vi "FrontPanel.vi"() -> ()   [LabVIEW 2013]
doc: "This VI controls the blindpanel type GHS-2T-1T-700 for a CryoFree DR. Automatization control is embedded in the blindpanel. Keys can be manipulated from within this VI."
uses:
  Write to PGSQL/FP to PGSQL/Typedefs/FP-cluster.ctl
  Lib/Lib.llb/ErrCodeStatusLkup.vi
  Lib/Lib.llb/Pfeiffer Vacuum.lvlib
  Lib/Lib.llb/MView.lvlib
  Lib/Lib.llb/Busy PopUp.lvlib
panel:
  out "VIRef":T1 {"Array DataType" format="%.0x"; "WaveForm Type" format="%.0x"; "RefNum Type" format="%.0x"; "DataType" format="%.0x"}
  out "ControlNames":string[](array[string])
  in  "Toolbar":enum32{"Page 1", "Page 2"}(tab)
  in  "Load config":bool
  in  "Save config":bool
  in  "Start":bool
  in  "Stop":bool
  out "V":string
  out "PT2 Data":dbl[](array[numeric])
  in  "Restart PT on Error?":bool
  in  "Attempts":u16=6
  in  "Time delay":u16=60 format="%.0f s"
  out "Error Log":string[][](table)
  in  "Error panel":enum32{"Page 1"}(tab)
  out "PT2 error":errorcluster
  out "MG error":errorcluster
  out "PT1 error":errorcluster
  out "FP error":errorcluster
  out "PT1 Data":dbl[](array[numeric])
  in  "Main Panel":enum32{"Page 1", "Page 2"}(tab)
  out "PC":sgl
  out "P1":sgl format="%.1f"
  out "P2":sgl format="%.1f"
  out "P3":sgl format="%.1f"
  out "P4":sgl format="%.1f"
  out "P5":sgl format="%.1f"
  out "P6":sgl format="%.1f"
  out "P7":sgl format="%.1f"
  out "Flow":sgl format="%#_4f"
  out "P5 alarm":bool
  out "Pstill (P8)":dbl format="%.1e"
  in  "Main Panel":T2(tab)
  out "String 2":string
  out "String 4":string
  out "String":string
  out "String 3":string
  out "Mode":u16(ring) items=["AUTO MODE OFF", "START", "CONDENSING 3He", "CONDENSING 4He", "NORMAL CIRCULATION", "RECOVERY OF THE MIXTURE", "RECOVERY: BLOCKAGE OR OVERPRESSURE"]
  out "FLOW":sgl format="%#_3f"
  out "P5":sgl
  out "P4":sgl
  out "P3":sgl
  out "P1":sgl
  out "P2":sgl
  out "3He":sgl(slide) min=0 max=2 scale=0.0..2000.0 scale format="%.2f"
  out "4He":sgl(slide) min=0 max=2 scale=0.0..2000.0 scale format="%.2f"
  out "Panel ID":string
  in  "FP type":enum32{"OLD", "NEW"}(tab)
  in  "Buttons":T3
  out "LEDs":T4
  in  "Buttons 2":T3
  out "LEDs 2":T5
  out "PC":sgl
  in  "PT Start 2":bool
  in  "PT_stop 2":bool
  in  "PT2 Plots Select":T6
  out "PT2 Status":cluster{"Time":dbl[], "Value":dbl[]}[](graph)
  in  "PT_ResetValues 2":bool
  out "PT Error Code 2":i32 caption="PT Error Code"
  out "PT Error 2":string="NO ERROR" caption="PT Error"
  out "P High":cluster{dbl, dbl, dbl, dbl}(slide) scale=150.0..450.0
  out "P Low":cluster{dbl, dbl, dbl, dbl}(slide) scale=0.0..300.0
  out "P_avg 2":cluster{"Low":dbl, "High":dbl} caption="Average pressure"
  out "Helium":cluster{dbl, dbl, dbl, dbl}(slide) scale=0.0..95.0
  out "Water In":cluster{dbl, dbl, dbl, dbl}(slide) scale=0.0..35.0
  out "Water Out":cluster{dbl, dbl, dbl, dbl}(slide) scale=0.0..60.0
  out "PT Status":u16(ring) items=["Compressor OFF", "Compressor ON", ""]
  out "Motor":cluster{dbl, dbl}(slide) scale=0.0..30.0
  out "Oil":cluster{dbl, dbl, dbl, dbl}(slide) scale=0.0..60.0
  in  "PT1 Plots Select":T6
  out "PT1 Status 2":cluster{"Time":dbl[], "Value":dbl[]}[](graph)
  out "P Low":cluster{dbl, dbl, dbl, dbl}(slide) scale=0.0..300.0
  out "P High":cluster{dbl, dbl, dbl, dbl}(slide) scale=150.0..450.0
  out "P_avg":cluster{"Low":dbl, "High":dbl} caption="Average pressure"
  out "Motor":cluster{dbl, dbl}(slide) scale=0.0..30.0
  out "Oil":cluster{dbl, dbl, dbl, dbl}(slide) scale=0.0..60.0
  out "Helium":cluster{dbl, dbl, dbl, dbl}(slide) scale=0.0..95.0
  out "Water Out":cluster{dbl, dbl, dbl, dbl}(slide) scale=0.0..60.0
  out "Water In":cluster{dbl, dbl, dbl, dbl}(slide) scale=0.0..35.0
  out "PT Error Code":i32
  out "PT Error":string="NO ERROR"
  in  "PT_ResetValues":bool
  in  "PT Start":bool
  in  "PT_stop":bool
  out "PT Status":u16(ring) items=["Compressor OFF", "Compressor ON", ""]
  in  "MG Plots Select":T6
  in  "FP Plots Select":T6
  out "MaxiGauge":cluster{"Time":dbl[], "Value":dbl[]}[](graph)
  out "Front Panel":cluster{"Time":dbl[], "Value":dbl[]}[](graph)
  in  "Boolean 2":bool
  out "PT2 port":u16
  out "PT1 port":u16
  out "MG port":refnum<visa-resource-name>="COM4" caption="Port number"
  out "FP port":refnum<visa-resource-name>="COM3" caption="Port number"
  out "ForceSave":bool
  in  "Button":u8
  out "SetControl":T7
  in  "S2":enum32{"Page 1"}(tab)
  in  "Reset Error 2":bool
  in  "S1":enum32{"Page 1"}(tab)
  in  "Reset Error":bool
  out "Cur Path":path
  in  "Side Panel":enum32{"Main", "Settings", "Advanced"}(tab)=enum."Settings"
  out "Maxigauge ID":string caption="ID"
  out "Panel response":string
  out "Sensors Status":T8={"String 8"="OK", "String 9"="OK", "String 10"="OK", "String 11"="OK", "String 12"="OK", "String 13"="OK"}
  in  "ADC scaling":T9={"P1"=2500.0, "P2"=2500.0, "P3"=2500.0, "P4"=2500.0, "P5"=2500.0, "P6"=2500.0, "P7"=2500.0, "Flow meter"=682.0, "PC"=10000.0} caption="Front panel ADC scaling factors" {"Flow meter" format="%#.4f"}
  in  "REC Settings":T10={"P6 low"=20, "P6 high"=1000, "P7 low"=20}
  in  "NCP5B Settings":cluster{"P6 low":u16}={"P6 low"=20}
  in  "NCP5 Settings":T10={"P6 low"=20, "P6 high"=1000, "P7 low"=20}
  in  "S1&2 Settings":cluster{"Enum":enum16{"OFF", "ON"}}
  in  "P5 Settings":cluster{"P6 low":u16, "P6 high":u16}={"P6 low"=20, "P6 high"=1000}
  out "REC limits":T11={"P5 warn"=20, "P5 rec"=20, "P5 res"=20}
  out "NCP5B limits":cluster{"P5 NC4":u16}={"P5 NC4"=20}
  out "NCP5 limits":T12={"P5 NC1"=20, "P5 NC2"=20, "P5 NC3"=20}
  out "S1&2 limits":cluster{"S1&S2":enum16{"OFF", "ON"}}
  out "P5 limits":cluster{"P5 C1":u16, "P5 C2":u16}={"P5 C1"=20, "P5 C2"=20}
  in  "P6&7 Settings":T13={"P6 low"=20, "P6 high"=1600, "P7 low"=20, "P7 high"=1610}
  out "P6&7 limits":T13={"P6 low"=20, "P6 high"=20, "P7 low"=20, "P7 high"=20}
  in  "SET VALUES":bool
  out "MG pressures":T14 {"Channel 1" format="%-7.2e mbar"; "Channel 1" format="%-7.2e mbar"; "Channel 1" format="%-7.2e mbar"; "Channel 1" format="%-7.2e mbar"; "Channel 1" format="%-7.2e mbar"; "Channel 1" format="%-7.2e mbar"}
  out "Cluster":T15={"String 2"="\"\"", "String 3"="", "String 4"="", "String 5"="", "String 6"="", "String 7"=""}
  in  "Log Options":T16={"Plot data "=TRUE, "Every1"=1.0, "Save to log"=TRUE, "Every  2"=1.0, "AVS_Path 2"=path "C:/LC Data/Data", "AVS_FName"="logFP", "Filename suffix"="_%Y-%m-%d-%H-%M-%S", "NewFevery"=7, "Time Units"=enum."Days", "Date Format"="%Y-%m-%d %H:%M:%S", "Averages"=4} caption="Data Logging \nOptions" {"Every  2" format="%#_g min"; "Every1" format="%#_g min"}
  in  "Configuration":T17={"FP port number"="COM3", "MG port number"="COM4", "PT1 Enabled?"=FALSE, "MG  channel P8"=65535, "Stop auto recovery if still is empty"=FALSE, "PT1 port number"="COM2", "MG Enabled?"=TRUE, "PT1 Address"=16, "S1 Enabled?"=FALSE, "S1 port"="COM2", "S2 Enabled?"=FALSE, "S2 port"="COM2", "Device address S1"=1, "Device address S2"=2, "PT1 Bauds"=115200, "PT2 Enabled?"=FALSE, "PT2 port number"="COM2", "PT2 Address"=16, "PT2 Bauds"=115200, "FP baud rate"=9600} {"PT2 Address" min=16 max=126 step=1; "MG  channel P8" items=["Channel 1", "Channel 2", "Channel 3", "Channel 4", "Channel 5", "Channel 6"]; "PT1 Address" min=16 max=126 step=1}
  in  "Type":enum32{"Wet", "CF"}(radio)=enum."CF"
  in  "Panel Layout":enum32{"OLD", "NEW"}(ring)=enum."NEW"
  out "RAW ADC Values 2":dbl[](array[numeric]) caption="Converted ADC Values"
  in  "SendCMD":bool caption="Send"
  out "Response":string
  in  "Command":string
  out "SP reached? 2":bool
  in  "Cond1":bool
  in  "Delay Time":u32=30 caption="For a time delay of" format="%.0f min"
  in  "MG  channel":u16(ring)=65535 caption="MaxiGauge" items=["Channel 1", "Channel 2", "Channel 3", "Channel 4", "Channel 5", "Channel 6"]
  out "SP reached? 3":bool
  in  "P threshold":dbl=0.0005 caption="<" format="%#_2g mbar"
  in  "Cond2":bool
  out "SP reached?":bool
  out "Delay Timer":u32=10 caption="Timer" format="%<%M:%S>t"
  in  "EnableAutoCond":bool caption="Start"
  out "VI path":string
  out "RAW ADC Values":i32[](array[numeric])
  in  "Autoconf":bool caption="Autoconfigure"
  out "MG Data":dbl[](array[numeric]) format="%.3e"
  out "FP Data":sgl[](array[numeric]) format="%.2f"
  out "FP Status bits":u32[](array[numeric])
  out "Attempts Counter":u16
  # "Error log"
  # "Front panel status"
  # "MaxiGauge status"
  # "Pulse Tube 1 status"
  # "Pulse Tube 2 status"
  # "Leiden Cryogenics"
  # "to \nair"
  # "N.C."
  # "from\novc"
  # "from\nivc"
  # "from still"
  # "to 3He\nin-1"
  # "to 3He\nin-2"
  # "P8"
  # "AUX 1"
  # "BYPASS"
  # "MIXTURE\nCOMPRESSOR"
  # "M2"
  # "P6"
  # "M3"
  # "M1"
  # "AUX PORT-1"
  # "P7"
  # "TRAP"
  # "AUX TRAP"
  # "To \nAir"
  # "From\nIVC"
  # "From Still"
  # "To 3He\nin-1"
  # "To 3He\nin-2"
  # "To \nAir"
  # "N.C."
  # "from\novc"
  # "from\nivc"
  # "from still"
  # "to 3He\nin-1"
  # "to 3He\nin-2"
  # "Leiden Cryogenics"
  # "to \nair"
  # "N.C."
  # "from\novc"
  # "from\nivc"
  # "from still"
  # "to 3He\nin-1"
  # "to 3He\nin-2"
  # "P8"
  # "M2"
  # "P6"
  # "M3"
  # "TRAP"
  # "AUX TRAP"
  # "M1"
  # "AUX PORT-1"
  # "P7"
  # "AUX 1"
  # "To \nAir"
  # "From\nIVC"
  # "From Still"
  # "To 3He\nin-1"
  # "to 3He\nin-1"
  # "To 3He\nin-2"
  # "to \nair"
  # "N.C."
  # "from\novc"
  # "from\nivc"
  # "from still"
  # "to 3He\nin-2"
  # "Pulse Tube 1"
  # "Pulse Tube 2"
  # "Front Panel"
  # "MaxiGauge"
  # "Turbo2 (S2)"
  # "Turbo1 (S1)"
  # "MaxiGauge"
  # "#"
  # "NAME"
  # "PRESSURE"
  # "STATUS"
  # "1"
  # "2"
  # "3"
  # "4"
  # "5"
  # "6"
  # "Automatic mode pressure limits"
  # "Warning: These values influence the operation of the GHS in automatic mode. Please refer to the operation manual and consult with Leiden Cryogenics before changing them."
  # "NAME"
  # "FW"
  # "NEW"
  # "DESCRIPTION"
  # "Stop condensing 4He"
  # "Stop recovering 4He"
  # "Stop condensing 3He"
  # "Stop recovering 3He"
  # "Condensing->open 12"
  # "Condensing->close 9/12"
  # "Condensing->run S1&S2"
  # "NC->open second line"
  # "NC->start MC"
  # "NC->open aux. trap"
  # "NC->stop MC, close 7"
  # "All->P5 alarm"
  # "All->switch to recovery"
  # "All->reset"
  # "Front panel ADC scaling factors"
  # "Data Logging and Plotting"
  # "Front Panel"
  # "MaxiGauge"
  # "Pulse Tube 1"
  # "Pulse Tube 2"
  # "Turbo 1 (S1) (Pfeiffer HiPACE only)"
  # "Turbo2 (S2) (Pfeiffer HiPACE only)"
  # "Automatic condensing"
  # "Start condensing when"
  # "and wait"
  # "Send command to Front Panel"
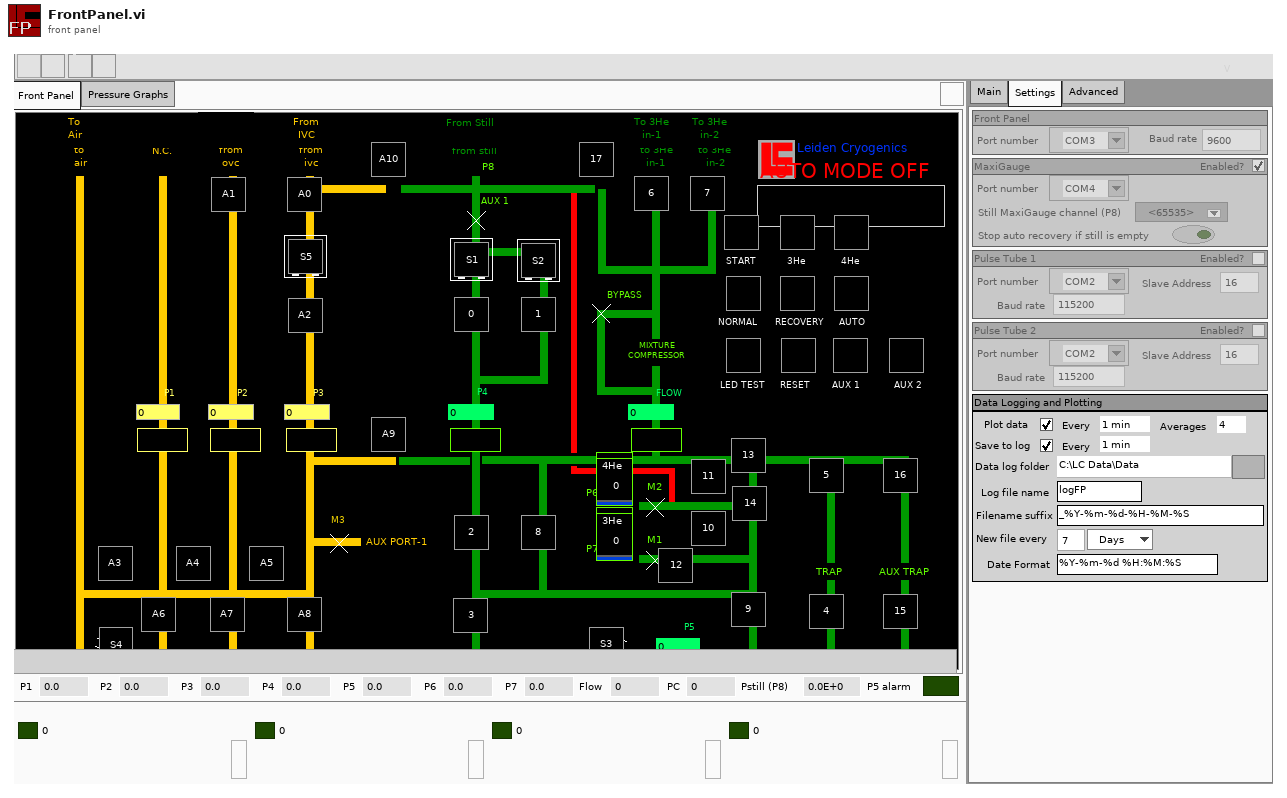
[diagram p1: front panel]
types:
  T1 = cluster{"Control Ref ID":refnum<vi>[], "Full Name":string[], "ClassID":enum16{"<Null>", "1", "2", "Generic", "Decoration", "Text", "Control", "ColorBox", "Boolean", "RefNum", "Variant", "Path", "ListBox", "Table", "Array", "Picture", "ActiveXContainer", "Numeric", "Digital", "NamedNumeric", "ColorRamp", "Slide", "GraphOrChart", "WaveformChart", "WaveformGraph", "IntensityChart", "IntensityGraph", "String", "IOName", "ComboBox", "Cluster", "Panel", "Knob", "NumWithScale", "Ring", "Enum", "GObject", "Plot", "Cursor", "NumericText", "Scale", "ColorScale", "GraphScale", "ColorGraphScale", "TypedRefNum", "OldKnobScale", "MCListbox", "MeasureData", "BVTag", "DAQName", "VISAName", "IVIName", "SlideScale", "TabControl", "Page", "TabArrayTabControl", "ConPane", "57", "58", "59", "60", "61", "62", "63", "64", "SubPanel", "TreeControl", "67", "68", "69", "70", "71", "72", "73", "74", "75", "SplitterBar"}[], "Short Name":string[], "DataType":enum8{"<Null>", "I8", "I16", "I32", "I64", "U8", "U16", "U32", "U64", "SGL", "DBL", "EXT", "CSG", "CDB", "CXT", "0x0F", "0x10", "0x11", "0x12", "0x13", "0x14", "Enum U8", "Enum U16", "Enum U32", "Enum U64", "SGL PQ", "DBL PQ", "EXT PQ", "CSG PQ", "CDB PQ", "CXT PQ", "0x1F", "0x20", "Boolean", "0x22", "0x23", "0x24", "0x25", "0x26", "0x27", "0x28", "0x29", "0x2A", "0x2B", "0x2C", "0x2D", "0x2E", "0x2F", "String", "0x31", "Path", "Pict", "0x34", "0x35", "0x36", "DAQ", "0x38", "0x39", "0x3A", "0x3B", "0x3C", "0x3D", "0x3E", "0x3F", "Array", "0x41", "0x42", "0x43", "0x44", "0x45", "0x46", "0x47", "0x48", "0x49", "0x4A", "0x4B", "0x4C", "0x4D", "0x4E", "0x4F", "Cluster", "0x51", "0x52", "Variant", "Waveform", "0x55", "0x56", "0x57", "0x58", "0x59", "0x5A", "0x5B", "0x5C", "0x5D", "0x5E", "0x5F", "0x60", "0x61", "0x62", "0x63", "0x64", "0x65", "0x66", "0x67", "0x68", "0x69", "0x6A", "0x6B", "0x6C", "0x6D", "0x6E", "0x6F", "Refnum"}[], "RefNum Type":enum8{"Generic", "Datalog File Refnum", "Byte Stream File Refnum", "Device Refnum", "Occurence Refnum", "TCP Connection Refnum", "VISA Refnum (Obsolete)", "Automation Renum", "VI Server Refnum", "Menu Refnum", "IVI Refnum (Obsolete)", "IMAQ Session", "0x0C", "Datasocket Refnum", "VISA Resource", "IVI Logical Name", "UDP Connection Refnum", "Notifier Refnum", "Queue Refnum", "IrDA Refnum", "Hardware Plugin Refnum", "Hardware Plugin Tag Refnum", "DAQmx Refnum", "Event Registration Refnum", ".NET Refnum", "User Event Refnum", "0x1A", "Event Callback", "0x1C", "0x1D", "Only Used Internal to LabVIEW", "Bluetooth", "Data Value References", "RT FIFO", "TDM Streaming"}[], "WaveForm Type":enum8{"<Not a Waveform Type>", "0x01", "Analog 16-bit signed", "Analog Double-Precision", "0x04", "Analog Single Precision", "Timestamp", "Digital Data", "Digital Waveform", "Dynamic Data", "Analog Extended-Precision", "Analog 8-bit unsigned", "Analog 16-bit unsigned", "Analog 32-bit unsigned", "Analog 8-bit signed", "Analog 32-bit signed", "Analog Complex Single-Precision", "Analog Complex Double-Precision", "Analog Complex Extended Precision", "Analog 64-bit signed", "Analog 64-bit unsigned"}[], "Parent":i32[], "Array DataType":enum8{"<Null>", "I8", "I16", "I32", "I64", "U8", "U16", "U32", "U64", "SGL", "DBL", "EXT", "CSG", "CDB", "CXT", "0x0F", "0x10", "0x11", "0x12", "0x13", "0x14", "Enum U8", "Enum U16", "Enum U32", "Enum U64", "SGL PQ", "DBL PQ", "EXT PQ", "CSG PQ", "CDB PQ", "CXT PQ", "0x1F", "0x20", "Boolean", "0x22", "0x23", "0x24", "0x25", "0x26", "0x27", "0x28", "0x29", "0x2A", "0x2B", "0x2C", "0x2D", "0x2E", "0x2F", "String", "0x31", "Path", "Pict", "0x34", "0x35", "0x36", "DAQ", "0x38", "0x39", "0x3A", "0x3B", "0x3C", "0x3D", "0x3E", "0x3F", "Array", "0x41", "0x42", "0x43", "0x44", "0x45", "0x46", "0x47", "0x48", "0x49", "0x4A", "0x4B", "0x4C", "0x4D", "0x4E", "0x4F", "Cluster", "0x51", "0x52", "Variant", "Waveform", "0x55", "0x56", "0x57", "0x58", "0x59", "0x5A", "0x5B", "0x5C", "0x5D", "0x5E", "0x5F", "0x60", "0x61", "0x62", "0x63", "0x64", "0x65", "0x66", "0x67", "0x68", "0x69", "0x6A", "0x6B", "0x6C", "0x6D", "0x6E", "0x6F", "Refnum"}[], "Owning VI":refnum<vi>[], "Active?":bool[]}
  T2 = enum32{"Front Panel", "PulseTube", "Pressure Graphs"}
  T3 = cluster{"baux2":bool, "bBypass":bool, "b15":bool, "b16":bool, "NC 0":bool, "baux1":bool, "b4":bool, "NC 1":bool, "b5":bool, "breset":bool, "NC 2":bool, "b9":bool, "b14":bool, "NC 3":bool, "b13":bool, "bledtest":bool, "NC 4":bool, "b12":bool, "b10":bool, "NC 5":bool, "b11":bool, "bA0":bool, "NC 9":bool, "b7":bool, "bS3":bool, "NC 12":bool, "b6":bool, "b17":bool, "NC 13":bool, "b8":bool, "b1":bool, "NC 14":bool, "bS2":bool, "b3":bool, "NC 15":bool, "b2":bool, "b0":bool, "NC 16":bool, "bS1":bool, "bA9":bool, "NC 17":bool, "bA8":bool, "bA2":bool, "NC 6":bool, "bs5":bool, "bA10":bool, "NC 7":bool, "bstart":bool, "bA5":bool, "NC 8":bool, "bA7":bool, "bA1":bool, "NC 10":bool, "bauto":bool, "bA4":bool, "NC 11":bool, "bA6":bool, "bS4":bool, "NC 18":bool, "bA3":bool, "b3he":bool, "b4he":bool, "bnorm":bool, "brecov":bool}
  T4 = cluster{"COMPR/AUX 2":bool, "BYPASS":bool, "15":bool, "16":bool, "NC 0":bool, "AUX 1":bool, "4":bool, "NC 1":bool, "5":bool, "RESET":bool, "NC 2":bool, "9":bool, "14":bool, "NC 3":bool, "13":bool, "LED TEST":bool, "NC 4":bool, "12":bool, "10":bool, "NC 5":bool, "11":bool, "A0":bool, "NC 12":bool, "7":bool, "S3":bool, "NC 13":bool, "6":bool, "17":bool, "NC 14":bool, "8":bool, "1":bool, "NC 15":bool, "S2":bool, "3":bool, "NC 16":bool, "2":bool, "0":bool, "NC 17":bool, "S1":bool, "A9":bool, "NC 6":bool, "A8":bool, "A2":bool, "NC 7":bool, "S5":bool, "A10":bool, "NC 8":bool, "START":bool, "A5":bool, "NC 9":bool, "A7":bool, "A1":bool, "NC 10":bool, "AUTO":bool, "A4":bool, "NC 11":bool, "A6":bool, "S4":bool, "NC 18":bool, "A3":bool, "3He":bool, "4He":bool, "NORMAL":bool, "RECOVERY":bool, "PT STATUS":bool}
  T5 = cluster{"COMPR/AUX 2":bool, "BYPASS":bool, "15":bool, "16":bool, "AUX 1":bool, "AUX 1":bool, "4":bool, "AUX 2":bool, "5":bool, "RESET":bool, "AUX 3":bool, "9":bool, "14":bool, "NC 3":bool, "13":bool, "LED TEST":bool, "NC 4":bool, "12":bool, "10":bool, "NC 5":bool, "11":bool, "A0":bool, "NC 12":bool, "7":bool, "S3":bool, "NC 13":bool, "6":bool, "17":bool, "NC 14":bool, "8":bool, "1":bool, "NC 15":bool, "S2":bool, "3":bool, "NC 16":bool, "2":bool, "0":bool, "NC 17":bool, "S1":bool, "A9":bool, "NC 6":bool, "A8":bool, "A2":bool, "NC 7":bool, "S5":bool, "A10":bool, "NC 8":bool, "START":bool, "A5":bool, "NC 9":bool, "A7":bool, "A1":bool, "NC 10":bool, "AUTO":bool, "A4":bool, "NC 11":bool, "A6":bool, "S4":bool, "NC 18":bool, "A3":bool, "3He":bool, "4He":bool, "NORMAL":bool, "RECOVERY":bool, "PT STATUS":bool}
  T6 = cluster{"Boolean":bool, "Boolean 2":bool, "Boolean 3":bool, "Boolean 4":bool, "Boolean 5":bool, "Boolean 6":bool, "Boolean 7":bool, "Boolean 8":bool}
  T7 = cluster{"Name":string, "Scalar":string, "Array":string[][]}
  T8 = cluster{"String 8":string, "String 9":string, "String 10":string, "String 11":string, "String 12":string, "String 13":string}
  T9 = cluster{"P1":dbl, "P2":dbl, "P3":dbl, "P4":dbl, "P5":dbl, "P6":dbl, "P7":dbl, "Flow meter":dbl, "PC":dbl}
  T10 = cluster{"P6 low":u16, "P6 high":u16, "P7 low":u16}
  T11 = cluster{"P5 warn":u16, "P5 rec":u16, "P5 res":u16}
  T12 = cluster{"P5 NC1":u16, "P5 NC2":u16, "P5 NC3":u16}
  T13 = cluster{"P6 low":u16, "P6 high":u16, "P7 low":u16, "P7 high":u16}
  T14 = cluster{"Channel 1":dbl, "Channel 1":dbl, "Channel 1":dbl, "Channel 1":dbl, "Channel 1":dbl, "Channel 1":dbl}
  T15 = cluster{"String 2":string, "String 3":string, "String 4":string, "String 5":string, "String 6":string, "String 7":string}
  T16 = cluster{"Plot data ":bool, "Every1":dbl, "Save to log":bool, "Every  2":dbl, "AVS_Path 2":path, "AVS_FName":string, "Filename suffix":string, "NewFevery":u32, "Time Units":enum16{"Minutes", "Hours", "Days"}, "Date Format":string, "Averages":i32}
  T17 = cluster{"FP port number":refnum<visa-resource-name>, "MG port number":refnum<visa-resource-name>, "PT1 Enabled?":bool, "MG  channel P8":u16, "Stop auto recovery if still is empty":bool, "PT1 port number":refnum<visa-resource-name>, "MG Enabled?":bool, "PT1 Address":u8, "S1 Enabled?":bool, "S1 port":refnum<visa-resource-name>, "S2 Enabled?":bool, "S2 port":refnum<visa-resource-name>, "Device address S1":u8, "Device address S2":u8, "PT1 Bauds":u32, "PT2 Enabled?":bool, "PT2 port number":refnum<visa-resource-name>, "PT2 Address":u8, "PT2 Bauds":u32, "FP baud rate":u32}
  T18 = cluster{"error":bool, "code":i32, "source":string}
  T19 = cluster{"Dict. Var":u16, "Description":string, "Values":i32[]}[]
  T20 = cluster{"[3]":dbl, "[3]":dbl, "[3]":dbl, "Values[3] 2":dbl}
  T21 = cluster{"[1]":dbl, "[1]":dbl, "[1]":dbl, "Values[1] 2":dbl}
  T22 = cluster{"Values[0]":dbl, "Values[0]":dbl, "Values[0]":dbl, "Values[0] 2":dbl}
  T23 = cluster{"error":bool, "code":i32, "error source":string}
  T24 = cluster{"sensor status info[0]":string, "sensor status info[1]":string, "sensor status info[2]":string, "sensor status info[3]":string, "sensor status info[4]":string, "sensor status info[5]":string}
  T25 = cluster{"Filterred[0]":dbl, "Filterred[1]":dbl, "Filterred[2]":dbl, "Filterred[3]":dbl, "Filterred[4]":dbl, "Filterred[5]":dbl}
  T26 = typedef "FP-cluster.ctl" = cluster{"FP Data":sgl[], "MG Data":dbl[], "PT Data":dbl[], "FP Status Bits":u32[], "Mode":u16}
  T27 = cluster{"FP Data[0]":sgl, "FP Data[1]":sgl, "FP Data[2]":sgl, "FP Data[3]":sgl, "FP Data[4]":sgl, "FP Data[5]":sgl, "FP Data[6]":sgl, "FP Data[7]":sgl, "FP Data[8]":sgl}
  T28 = enum32{"Page Enabled", "Page Disabled", "Page Disabled & Grayed"}
  T29 = enum32{"invalid app kind", "Development System", "Run Time System", "Student Edition", "Embedded LabVIEW", "Evaluation", "Custom"}
  T30 = cluster{"array of 4 x 16 bit unsigned[0]":u16, "array of 4 x 16 bit unsigned[1]":u16, "array of 4 x 16 bit unsigned[2]":u16, "array of 4 x 16 bit unsigned[3]":u16}
  T31 = cluster{"array of 2 x 16 bit unsigned[0]":u16, "array of 2 x 16 bit unsigned[1]":u16}
  T32 = cluster{"array of 3 x 16 bit unsigned[0]":u16, "array of 3 x 16 bit unsigned[1]":u16, "array of 3 x 16 bit unsigned[2]":u16}
  T33 = cluster{"Array[0]":string, "Array[1]":string, "Array[2]":string, "Array[3]":string, "Array[4]":string, "Array[5]":string}
  T34 = typedef "LVRectTypeDef.ctl" = cluster{"Left":i16, "Top":i16, "Right":i16, "Bottom":i16}
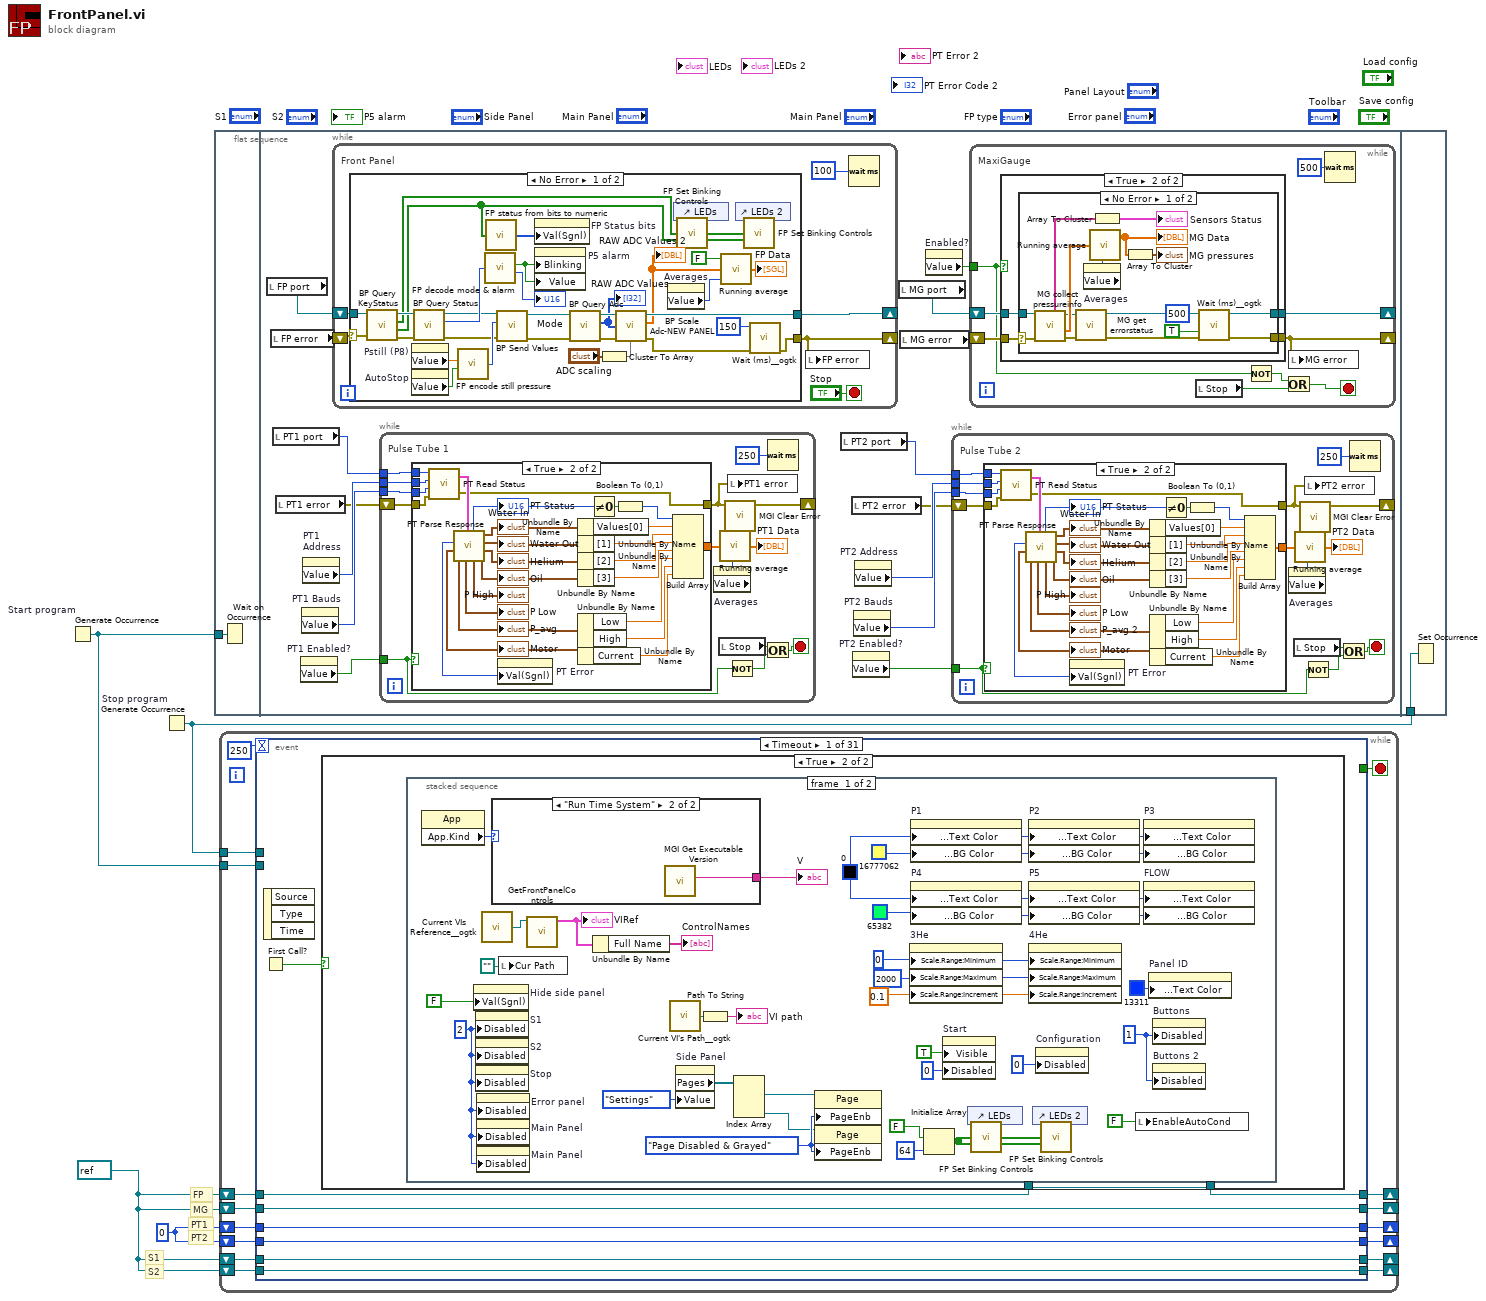
[diagram p0: block diagram]
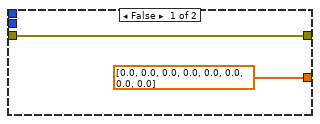
[diagram p2: hidden frame]
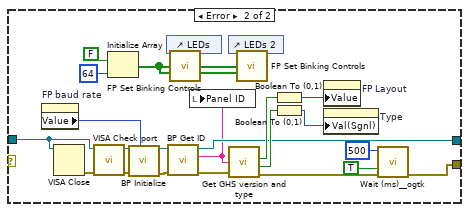
[diagram p3: hidden frame]
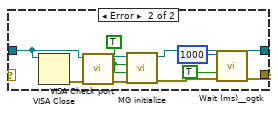
[diagram p5: hidden frame]
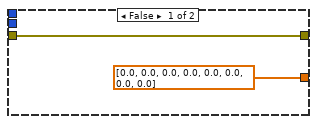
[diagram p6: hidden frame]
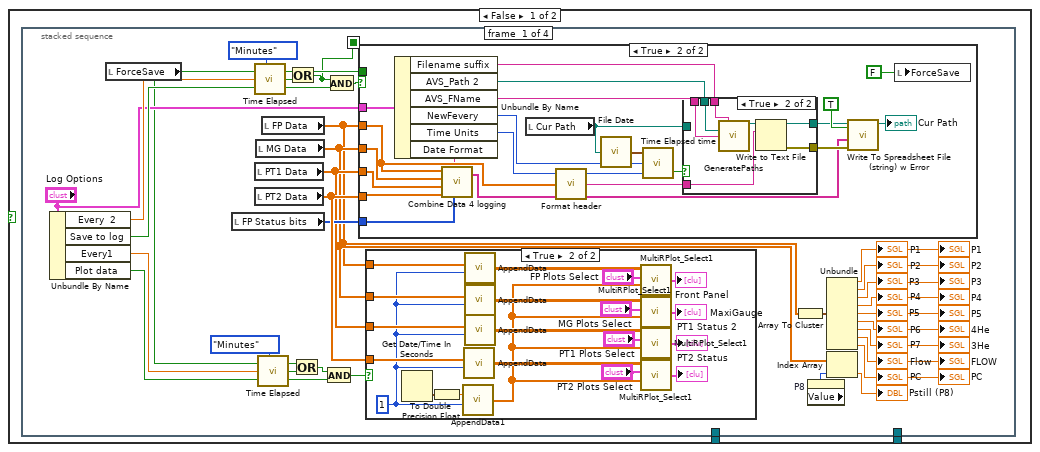
[diagram p7: hidden frame]
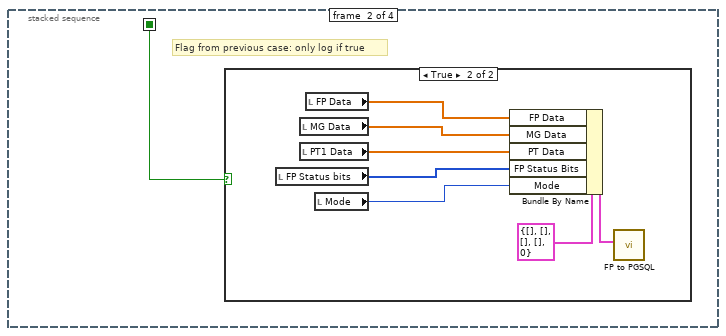
[diagram p11: hidden frame]
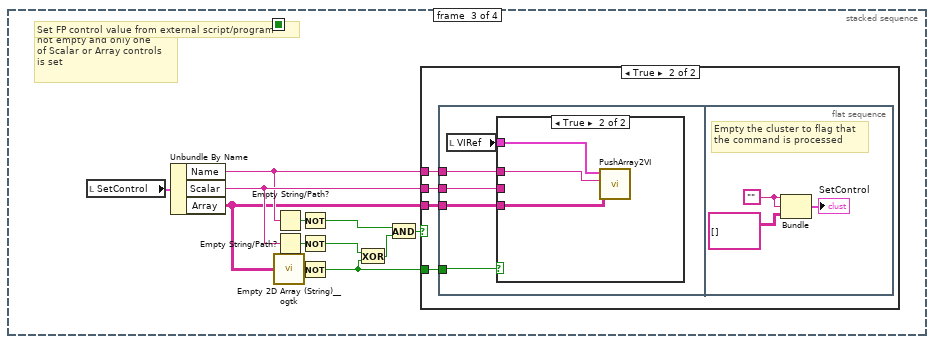
[diagram p13: hidden frame]
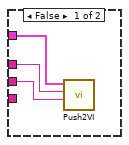
[diagram p15: hidden frame]
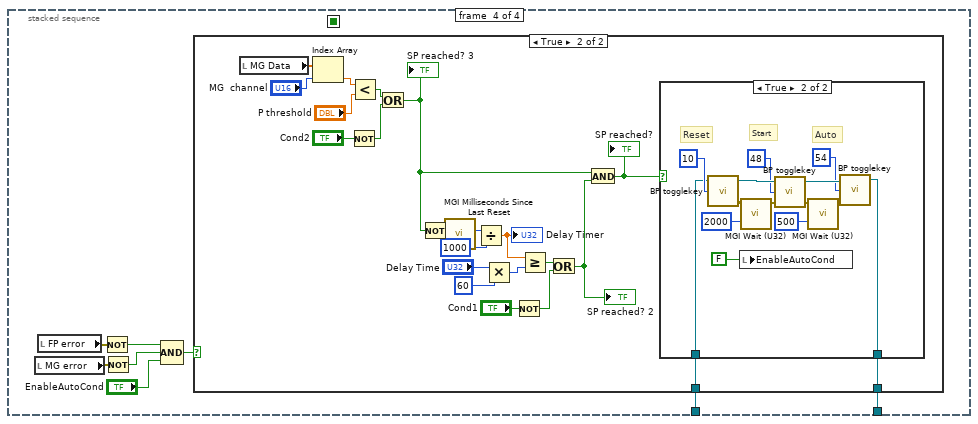
[diagram p16: hidden frame]
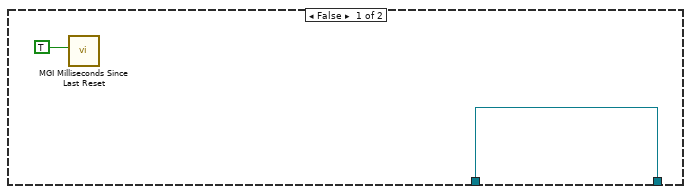
[diagram p17: hidden frame]
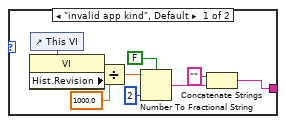
[diagram p19: hidden frame]
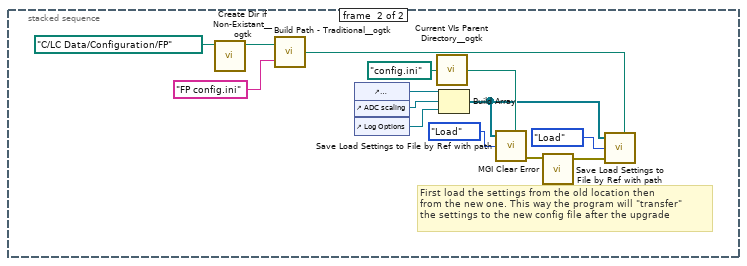
[diagram p20: hidden frame]
diagram:
  w1 = u8 0 ("x+1")
  w2 = refnum<visa-resource-name> refnum ("PT port")
  # "S2"
  # "S1"
  # "MG"
  # "PT1"
  # "PT2"
  # "FP"
  n1 = Generate Occurrence "Start program"() -> (w4:refnum<k4>)
  n2 = Generate Occurrence "Stop program"() -> (w3:refnum<k4>)
  n3 = flat-sequence {
    tunnel: w4 -> [w5]
    tunnel: w3 -> [w204]
    frame #0 {
      n4 = Wait on Occurrence(2:w5) -> ()  [unwired: 2 in, 1 out]
    }
    frame #1 {
      n5 = local read "FP port"() -> (w11:refnum<visa-resource-name>)
      n6 = local read "FP error"() -> (w16:errorcluster)
      n7 = local read "PT1 port"() -> (w7:u16)
      n8 = local read "PT1 error"() -> (w8:errorcluster)
      n9 = property on="PT1 Enabled?" class="Bool (strict)"() -> ("Value"=w19:bool)  [unwired: 2 in, 2 out]
      n10 = property on="PT1 Bauds" class="DigNum (strict)"() -> ("Value"=w17:u32)  [unwired: 2 in, 2 out]
      n11 = property on="PT1 \nAddress" class="DigNum (strict)"() -> ("Value"=w20:u8)  [unwired: 2 in, 2 out]
      n12 = while {
        shift-right: [w66] -> _
        shift-left: w16 -> [w67]
        shift-right: [w64] -> _
        shift-left: w11 -> [w65]
        stop <- "Stop" stop-if-true
        # "Front Panel"
        n13 = case shown="No Error" w67 {
          selector: w67 -> [w97 _]
          tunnel: [w78 w111] -> w64
          tunnel: [w76 w109] -> w66
          tunnel: w65 -> [w98 w112]
          frame No Error {
            n14 = call "BP Query KeyStatus.vi"("error in"=w97, "FrontPanel port"=w98) -> ("error out"=w86:T18, "Button states"=w69:bool[], "Blinking States"=w70:bool[], "FrontPanel port"=w87:refnum<visa-resource-name>)  [unwired: 2 in]
            n15 = property on="Pstill (P8)" class="DigNum (strict)"() -> ("Value"=w88:dbl)  [unwired: 2 in, 2 out]
            n16 = property on="AutoStop" class="Bool (strict)"() -> ("Value"=w89:bool)  [unwired: 2 in, 2 out]
            n17 = call "BP Query Status.vi"("error in"=w86, "FrontPanel port"=w87) -> ("error out"=w91:T18, "status word (32 bit unsigned)"=w94:u32, "FrontPanel port"=w92:refnum<visa-resource-name>)  [unwired: 3 in]
            n18 = call "FP encode still pressure.vi"("Value 2"=w89, "Value"=w88) -> ("Numeric"=w93:u16)  [unwired: 4 in]
            n19 = call "FP decode mode & alarm.vi"("status word (32 bit unsigned)"=w94) -> ("Boolean"=w90:bool, "Numeric"=→"Mode":u32)  [unwired: 4 in]
            n20 = call "FP status from bits to numeric.vi"("FP Status bits"=w69) -> ("FP status number"=w96:u32[])  [unwired: 4 in]
            n21 = call "BP Send Values.vi"("error in"=w91, "value to send"=w93, "FrontPanel port"=w92) -> ("error out"=w80:T18, "FrontPanel port"=w81:refnum<visa-resource-name>)  [unwired: 3 in]
            n22 = property on="FP Status bits" class="Arr (strict)"("Val(Sgnl)"=w96) -> ()  [unwired: 2 in, 2 out]
            n23 = property on="P5 alarm" class="Bool (strict)"("Blinking"=w90, "Value"=w90) -> ()  [unwired: 2 in, 2 out]
            n24 = call "BP Query Adc.vi"("error in"=w80, "FrontPanel port"=w81) -> ("error out"=w77:T18, "array of 8(9) x 16 bit signed"=w72:i32[], "FrontPanel port"=w78:refnum<visa-resource-name>)  [unwired: 3 in]
            "RAW ADC Values" <- w72
            n25 = Cluster To Array(cluster="ADC scaling") -> (array=w79:dbl[])
            n26 = call "BP Scale Adc-NEW PANEL.vi"("input array scaling factors,8(9) x 16 bit uint"=w79, "input array 8(9) x 16bit uint"=w72) -> ("output array 8(9) x single prec. incl flow"=w71:sgl[])  [unwired: 4 in, 1 out]
            "RAW ADC Values 2" <- w71
            n27 = property on="Averages" class="DigNum (strict)"() -> ("Value"=w85:i32)  [unwired: 2 in, 2 out]
            n28 = control-ref of="LEDs"() -> (w74:refnum<vi>)
            n29 = call "FP Set Binking Controls.vi"("Cluster in"=w74, "Array of blinking states"=w70, "Array of relais states"=w69) -> ()  [unwired: 13 in]
            n30 = call "Running average.vi"("Window Size"=w85, "New values"=w71, "Filter Zeroes? (T)"=FALSE) -> ("Filterred"=→"FP Data":dbl[])  [unwired: 1 in]
            n31 = control-ref of="LEDs 2"() -> (w73:refnum<vi>)
            n32 = call "FP Set Binking Controls.vi"("Cluster in"=w73, "Array of blinking states"=w70, "Array of relais states"=w69) -> ()  [unwired: 13 in]
            n33 = call "Wait (ms)__ogtk.vi"("error in (no error)"=w77, "milliseconds to wait"=u32 150) -> ("error out"=w76:errorcluster)  [unwired: 8 in, 1 out]
          }
          frame Error {
            n34 = property on="FP baud rate" class="DigNum (strict)"() -> ("Value"=w104:u32)  [unwired: 2 in, 2 out]
            n35 = VISA Close(VISA resource name=w112) -> (error out=w121:errorcluster)  [unwired: 1 in]
            n36 = call "VISA Check port.vi"("error in (no error)"=w121, "VISA Resource Name in"=w112) -> ("error out"=w120:errorcluster, "VISA Resource Name out"=w119:refnum<visa-resource-name>)  [unwired: 8 in]
            n37 = Initialize Array(FALSE, 64 ("dimension size")) -> (w99:bool[])
            n38 = call "BP Initialize.vi"("FP baud rate"=w104, "error in (no error)"=w120, "FrontPanel port"=w119) -> ("error out"=w118:errorcluster, "FrontPanel port"=w117:refnum<visa-resource-name>)  [unwired: 4 in]
            n39 = control-ref of="LEDs"() -> (w101:refnum<vi>)
            n40 = call "BP Get ID.vi"("error in (no error)"=w118, "FrontPanel port"=w117) -> ("error out"=w106:errorcluster, "Device ID string"=w110:string, "FrontPanel port"=w111:refnum<visa-resource-name>)  [unwired: 6 in, 1 out]
            n41 = call "FP Set Binking Controls.vi"("Cluster in"=w101, "Array of blinking states"=w99, "Array of relais states"=w99) -> ()  [unwired: 13 in]
            n42 = local write "Panel ID"(w110) -> ()
            n43 = control-ref of="LEDs 2"() -> (w100:refnum<vi>)
            n44 = call "Get GHS version and type.vi"("ID string"=w110, "error in (no error)"=w106) -> ("Panel Version"=w113:bool, "System Type"=w115:bool, "error out"=w105:errorcluster)  [unwired: 4 in]
            n45 = call "FP Set Binking Controls.vi"("Cluster in"=w100, "Array of blinking states"=w99, "Array of relais states"=w99) -> ()  [unwired: 13 in]
            n46 = Boolean To (0,1)(Boolean=w113) -> (0, 1=w114:i16)
            n47 = Boolean To (0,1)(Boolean=w115) -> (0, 1=w116:i16)
            n48 = property on="FP Layout" class="TabCtl (strict)"("Value"=w114) -> ()  [unwired: 2 in, 2 out]
            n49 = property on="Type" class="RadioBtnsControl (strict)"("Val(Sgnl)"=w116) -> ()  [unwired: 2 in, 2 out]
            n50 = call "Wait (ms)__ogtk.vi"("error in (no error)"=w105, "Wait on Error (FALSE)"=TRUE, "milliseconds to wait"=u32 500) -> ("error out"=w109:errorcluster)  [unwired: 7 in, 1 out]
          }
        }
        n51 = local write "FP error"(w66) -> ()
        n52 = Wait (ms)(milliseconds to wait=u32 100) -> ()  [unwired: 1 out]
      }
      n53 = while {
        tunnel: w7 -> [w174]
        tunnel: w20 -> [w173]
        tunnel: w19 -> [w164]
        tunnel: w17 -> [w170]
        shift-right: [w163] -> _
        shift-left: w8 -> [w169]
        stop <- w167 stop-if-true
        # "Pulse Tube 1"
        n54 = case shown="True" w164 {
          tunnel: [dbl[] [0.0, 0.0, 0.0, 0.0, 0.0, 0.0, 0.0, 0.0] w191] -> w175
          tunnel: w174 -> [_ w190]
          tunnel: w169 -> [w176 w189]
          tunnel: w173 -> [_ w188]
          tunnel: w170 -> [_ w183]
          tunnel: [w176 w182] -> w162
          frame False {
          }
          frame True {
            n55 = call "PT Read Status.vi"("error in (no error)"=w189, "Baud"=w183, "Slave Address"=w188, "Com Port #"=w190) -> ("error out"=w182:errorcluster, "Response"=w192:T19)
            n56 = call "PT Parse Response.vi"("Response"=w192) -> ("Oil temp"=w197:T20, "He temp"=w196:cluster{"[2]":dbl, "[2]":dbl, "[2]":dbl, dbl}, "Out water temp"=w195:T21, "In water temp"=w194:T22, "P_high"=→"P High":cluster{"[0]":dbl, "[0]":dbl, "[0]":dbl, dbl}, "Numeric"=w201:i32, "P_low"=→"P Low":cluster{"[1]":dbl, "[1]":dbl, "[1]":dbl, dbl}, "Average pressure"=w187:cluster{"Low":dbl, "High":dbl}, "Current"=w181:cluster{"Current":dbl, "Threshold":dbl}, "PT Error"=w193:i32)  [unwired: 1 in]
            "Oil" <- w197
            "Motor" <- w181
            "PT Status" <- w201
            "Water Out" <- w195
            "Water In" <- w194
            "Helium" <- w196
            "P_avg" <- w187
            n57 = property on="PT Error" class="DigNum (strict)"("Val(Sgnl)"=w193) -> ()  [unwired: 2 in, 2 out]
            n58 = Unbundle By Name(w194) -> ("Values[0]"=w184:dbl)
            n59 = Unbundle By Name(w195) -> ("[1]"=w200:dbl)
            n60 = Unbundle By Name(w196) -> ("[2]"=w199:dbl)
            n61 = Unbundle By Name(w197) -> ("[3]"=w198:dbl)
            n62 = Unbundle By Name(w187) -> ("Low"=w186:dbl, "High"=w185:dbl)
            n63 = Unbundle By Name(w181) -> ("Current"=w180:dbl)
            n64 = Not Equal To 0?(x=w201) -> (x != 0?=w202:bool)
            n65 = Boolean To (0,1)(Boolean=w202) -> (0, 1=w203:i16)
            n66 = Build Array(w203, w184, w200, w199, w198, w186, w185, w180) -> (w191:dbl[])
          }
        }
        n67 = property on="Averages" class="DigNum (strict)"() -> ("Value"=w172:i32)  [unwired: 2 in, 2 out]
        n68 = local read "Stop"() -> (w166:bool)
        n69 = call "Running average.vi"("Window Size"=w172, "New values"=w175) -> ("Filterred"=→"PT1 Data":dbl[])  [unwired: 2 in]
        n70 = call "MGI Clear Error.vi"("Error In"=w162) -> ("Error Out"=w163:errorcluster)  [unwired: 6 in]
        n71 = Not(x=w164) -> (.not. x?=w165:bool)
        n72 = local write "PT1 error"(w162) -> ()
        n73 = Or(x=w166, y=w165) -> (x .or. y?=w167:bool)
        n74 = Wait (ms)(milliseconds to wait=u32 250) -> ()  [unwired: 1 out]
      }
      n75 = local read "PT2 port"() -> (w6:u16)
      n76 = local read "PT2 error"() -> (w9:errorcluster)
      n77 = property on="PT2 Enabled?" class="Bool (strict)"() -> ("Value"=w13:bool)  [unwired: 2 in, 2 out]
      n78 = property on="PT2 Bauds" class="DigNum (strict)"() -> ("Value"=w12:u32)  [unwired: 2 in, 2 out]
      n79 = property on="PT2 Address" class="DigNum (strict)"() -> ("Value"=w14:u8)  [unwired: 2 in, 2 out]
      n80 = local read "MG port"() -> (w10:refnum<visa-resource-name>)
      n81 = local read "MG error"() -> (w15:errorcluster)
      n82 = property on="Enabled?" class="Bool (strict)"() -> ("Value"=w18:bool)  [unwired: 2 in, 2 out]
      n83 = while {
        tunnel: w6 -> [w33]
        tunnel: w14 -> [w32]
        tunnel: w13 -> [w23]
        tunnel: w12 -> [w29]
        shift-right: [w22] -> _
        shift-left: w9 -> [w28]
        stop <- w26 stop-if-true
        # "Pulse Tube 2"
        n84 = case shown="True" w23 {
          tunnel: [dbl[] [0.0, 0.0, 0.0, 0.0, 0.0, 0.0, 0.0, 0.0] w50] -> w34
          tunnel: w33 -> [_ w49]
          tunnel: w28 -> [w35 w48]
          tunnel: w32 -> [_ w47]
          tunnel: w29 -> [_ w42]
          tunnel: [w35 w41] -> w21
          frame False {
          }
          frame True {
            n85 = call "PT Read Status.vi"("error in (no error)"=w48, "Baud"=w42, "Slave Address"=w47, "Com Port #"=w49) -> ("error out"=w41:errorcluster, "Response"=w51:T19)
            n86 = call "PT Parse Response.vi"("Response"=w51) -> ("Oil temp"=w56:T20, "He temp"=w55:cluster{"[2]":dbl, "[2]":dbl, "[2]":dbl, dbl}, "Out water temp"=w54:T21, "In water temp"=w53:T22, "P_high"=→"P High":cluster{"[0]":dbl, "[0]":dbl, "[0]":dbl, dbl}, "Numeric"=w60:i32, "P_low"=→"P Low":cluster{"[1]":dbl, "[1]":dbl, "[1]":dbl, dbl}, "Average pressure"=w46:cluster{"Low":dbl, "High":dbl}, "Current"=w40:cluster{"Current":dbl, "Threshold":dbl}, "PT Error"=w52:i32)  [unwired: 1 in]
            "Oil" <- w56
            "Motor" <- w40
            "PT Status" <- w60
            "Water Out" <- w54
            "Water In" <- w53
            "Helium" <- w55
            "P_avg 2" <- w46
            n87 = property on="PT Error" class="DigNum (strict)"("Val(Sgnl)"=w52) -> ()  [unwired: 2 in, 2 out]
            n88 = Unbundle By Name(w53) -> ("Values[0]"=w43:dbl)
            n89 = Unbundle By Name(w54) -> ("[1]"=w59:dbl)
            n90 = Unbundle By Name(w55) -> ("[2]"=w58:dbl)
            n91 = Unbundle By Name(w56) -> ("[3]"=w57:dbl)
            n92 = Unbundle By Name(w46) -> ("Low"=w45:dbl, "High"=w44:dbl)
            n93 = Unbundle By Name(w40) -> ("Current"=w39:dbl)
            n94 = Not Equal To 0?(x=w60) -> (x != 0?=w61:bool)
            n95 = Boolean To (0,1)(Boolean=w61) -> (0, 1=w62:i16)
            n96 = Build Array(w62, w43, w59, w58, w57, w45, w44, w39) -> (w50:dbl[])
          }
        }
        n97 = property on="Averages" class="DigNum (strict)"() -> ("Value"=w31:i32)  [unwired: 2 in, 2 out]
        n98 = local read "Stop"() -> (w25:bool)
        n99 = call "Running average.vi"("Window Size"=w31, "New values"=w34) -> ("Filterred"=→"PT2 Data":dbl[])  [unwired: 2 in]
        n100 = call "MGI Clear Error.vi"("Error In"=w21) -> ("Error Out"=w22:errorcluster)  [unwired: 6 in]
        n101 = Not(x=w23) -> (.not. x?=w24:bool)
        n102 = local write "PT2 error"(w21) -> ()
        n103 = Or(x=w25, y=w24) -> (x .or. y?=w26:bool)
        n104 = Wait (ms)(milliseconds to wait=u32 250) -> ()  [unwired: 1 out]
      }
      n105 = while {
        tunnel: w18 -> [w123]
        shift-right: [w127] -> _
        shift-left: w15 -> [w126]
        shift-right: [w125] -> _
        shift-left: w10 -> [w128]
        stop <- w124 stop-if-true
        # "MaxiGauge"
        n106 = case shown="True" w123 {
          tunnel: w128 -> [w132 w136]
          tunnel: [w131 w135] -> w127
          tunnel: w126 -> [w131 w134]
          tunnel: [w132 w133] -> w125
          frame False {
          }
          frame True {
            n107 = case shown="No Error" w134 {
              selector: w134 -> [w143 _]
              tunnel: w136 -> [w151 w161]
              tunnel: [w137 w152] -> w135
              tunnel: [w150 w160] -> w133
              frame No Error {
                n108 = call "MG collect pressureinfo.vi"("error in"=w143, "MaxiGauge port"=w151) -> ("error out"=w148:T23, "sensor values"=w146:dbl[], "MaxiGauge port"=w142:refnum<visa-resource-name>, "sensor status info"=w141:string[])  [unwired: 4 in, 2 out]
                n109 = call "MG get errorstatus.vi"("error in"=w148, "MaxiGauge port"=w142) -> ("error out"=w138:T23, "MaxiGauge port"=w150:refnum<visa-resource-name>)  [unwired: 2 in, 2 out]
                n110 = property on="Averages" class="DigNum (strict)"() -> ("Value"=w145:i32)  [unwired: 2 in, 2 out]
                n111 = call "Running average.vi"("Window Size"=w145, "New values"=w146) -> ("Filterred"=w144:dbl[])  [unwired: 2 in]
                "MG Data" <- w144
                n112 = Array To Cluster(array=w141) -> (cluster=→"Sensors Status":T24)
                n113 = Array To Cluster(array=w144) -> (cluster=→"MG pressures":T25)
                n114 = call "Wait (ms)__ogtk.vi"("error in (no error)"=w138, "Wait on Error (FALSE)"=TRUE, "milliseconds to wait"=u32 500) -> ("error out"=w137:errorcluster)  [unwired: 7 in, 1 out]
              }
              frame Error {
                w156 = TRUE ("ID query")
                n115 = VISA Close(VISA resource name=w161) -> (error out=w159:errorcluster)  [unwired: 1 in]
                n116 = call "VISA Check port.vi"("error in (no error)"=w159, "VISA Resource Name in"=w161) -> ("error out"=w158:errorcluster, "VISA Resource Name out"=w157:refnum<visa-resource-name>)  [unwired: 8 in]
                n117 = call "MG initialize.vi"("error in (no error)"=w158, "MG query errorstatus"=w156, "ID query"=w156, "MaxiGauge port"=w157) -> ("error out"=w153:errorcluster, "MaxiGauge port"=w160:refnum<visa-resource-name>)  [unwired: 2 in, 1 out]
                n118 = call "Wait (ms)__ogtk.vi"("error in (no error)"=w153, "Wait on Error (FALSE)"=TRUE, "milliseconds to wait"=u32 1000) -> ("error out"=w152:errorcluster)  [unwired: 7 in, 1 out]
              }
            }
          }
        }
        n119 = local read "Stop"() -> (w129:bool)
        n120 = Not(x=w123) -> (.not. x?=w122:bool)
        n121 = Or(x=w122, y=w129) -> (x .or. y?=w124:bool)
        n122 = local write "MG error"(w127) -> ()
        n123 = Wait (ms)(milliseconds to wait=u32 500) -> ()  [unwired: 1 out]
      }
    }
    frame #2 {
      n124 = Set Occurrence(w204) -> ()
    }
  }
  n125 = while {
    shift-right: [w212] -> _
    shift-left: w2 -> [w218]
    shift-right: [w216] -> _
    shift-left: w2 -> [w217]
    tunnel: w4 -> [w215]
    shift-right: [w213] -> _
    shift-left: w1 -> [w214]
    shift-right: [w209] -> _
    shift-left: w2 -> [w211]
    shift-right: [w208] -> _
    shift-left: w2 -> [w210]
    tunnel: w3 -> [w207]
    shift-right: [w205] -> _
    shift-left: w1 -> [w206]
    stop <- w220 stop-if-true
    n126 = event shown="[0] Timeout" {
      selector: _ -> [_ _ _ _ _ _ _ _ _ _ _ _ _ _ _ _ _ _ _ _ _ _ _ _ _ _ _ _ _ _ _]
      dyn-events: _ -> [_ _ _ _ _ _ _ _ _ _ _ _ _ _ _ _ _ _ _ _ _ _ _ _ _ _ _ _ _ _ _]
      timeout: 250 -> [_ _ _ _ _ _ _ _ _ _ _ _ _ _ _ _ _ _ _ _ _ _ _ _ _ _ _ _ _ _ _]
      tunnel: [_ _ TRUE _ _ _ _ _ _ _ _ _ _ _ _ _ _ _ _ _ _ _ _ _ _ _ _ _ _ _ _] -> w220
      tunnel: w218 -> [w221 w463 w629 w661 w670 w679 w688 w700 w731 w740 w746 w759 w773 w777 w882 w891 w904 w920 w935 w941 w961 w971 w986 w993 w1001 w1009 w1020 w1037 w1043 w1066 w1071]
      tunnel: w217 -> [w224 w465 w628 w660 w669 w678 w687 w699 w730 w739 w744 w757 w771 w781 w881 w890 w905 w919 w934 w940 w960 w970 w985 w994 w1002 w1008 w1019 w1036 w1041 w1065 w1074]
      tunnel: [w224 w464 w615 w660 w669 w678 w687 w699 w730 w739 w744 w757 w771 w781 w881 w890 w903 w919 w934 w940 w960 w970 w985 w994 w1002 w1008 w1019 w1036 w1041 w1065 w1074] -> w216
      tunnel: w215 -> [_ w461 _ _ _ _ _ _ _ _ _ _ _ _ _ _ _ _ _ _ _ _ _ _ _ _ _ _ _ _ _]
      tunnel: w214 -> [w227 w453 _ w659 w668 w677 w686 w696 w729 w738 w752 w764 w775 w780 w880 w892 _ w921 w933 w942 w959 w972 w982 w992 w1000 w1010 w1021 w1035 w1042 w1064 w1076]
      tunnel: [w227 w455 w614 w659 w668 w677 w686 w696 w729 w738 w752 w764 w775 w780 w880 w892 w893 w921 w933 w942 w959 w972 w982 w992 w1000 w1010 w1021 w1035 w1042 w1064 w1076] -> w213
      tunnel: [w222 w462 w615 w661 w670 w679 w688 w700 w731 w740 w745 w758 w772 w776 w882 w891 w906 w920 w935 w941 w961 w971 w986 w993 w1001 w1009 w1020 w1037 w1043 w1066 w1070] -> w212
      tunnel: w211 -> [w226 w460 w627 w658 w667 w676 w685 w692 w728 w737 w743 w756 w770 w779 w879 w889 w902 w918 w931 w939 w958 w969 w984 w996 w1003 w1007 w1018 w1033 w1040 w1062 w1073]
      tunnel: w210 -> [w225 w459 w626 w657 w666 w675 w684 w691 w727 w736 w742 w755 w769 w778 w878 w888 w900 w917 w930 w938 w957 w968 w983 w995 w1004 w1006 w1017 w1032 w1039 w1061 w1072]
      tunnel: [w226 w458 w615 w658 w667 w676 w685 w692 w728 w737 w743 w756 w770 w779 w879 w889 w901 w918 w931 w939 w958 w969 w984 w990 w1003 w1007 w1018 w1033 w1040 w1062 w1073] -> w209
      tunnel: [w225 w457 w615 w657 w666 w675 w684 w691 w727 w736 w742 w755 w769 w778 w878 w888 w899 w917 w930 w938 w957 w968 w983 w995 w998 w1006 w1017 w1032 w1039 w1061 w1072] -> w208
      tunnel: w207 -> [_ _ w625 _ _ _ _ _ _ _ _ _ _ _ _ _ _ _ _ _ _ _ _ _ _ _ _ _ _ _ _]
      tunnel: w206 -> [w223 w456 _ w656 w665 w674 w683 w690 w726 w735 w751 w765 w774 w783 w877 w887 _ w908 w932 w937 w947 w964 w981 w989 w997 w1005 w1016 w1034 w1038 w1063 w1075]
      tunnel: [w223 w454 w614 w656 w665 w674 w683 w690 w726 w735 w751 w765 w774 w783 w877 w887 w895 w908 w932 w937 w947 w964 w981 w989 w997 w1005 w1016 w1034 w1038 w1063 w1075] -> w205
      event Timeout {
        n127 = First Call?() -> (First Call?: T/F=w228:bool)
        n128 = event-data() -> ()  [unwired: 1 in, 3 out]
        n129 = case shown="True" w228 {
          tunnel: w221 -> [w230 w396]
          tunnel: [w229 w396] -> w222
          frame False {
            n130 = stacked-sequence {
              seq-local: [w231 _ _ _] -> [_ w311 _ _]
              tunnel: w230 -> [_ _ _ w356]
              tunnel: [_ _ _ w355] -> w229
              frame #0 {
                n131 = Unbundle By Name("Log Options") -> ("Every  2"=w248:dbl, "Save to log"=w249:bool, "Every1"=w240:dbl, "Plot data"=w250:bool)
                n132 = local read "ForceSave"() -> (w241:bool)
                n133 = local read "FP Status bits"() -> (w236:u32[])
                n134 = call "Time Elapsed.vi"("Every"=w248, "Time Units"=enum16{"Minutes", "Hours", "Days"}."Minutes") -> ("Triggered?"=w244:bool)  [unwired: 1 in]
                n135 = local read "PT1 Data"() -> (w235:dbl[])
                n136 = local read "PT2 Data"() -> (w239:dbl[])
                n137 = local read "MG Data"() -> (w234:dbl[])
                n138 = call "Time Elapsed.vi"("Every"=w240, "Time Units"=enum16{"Minutes", "Hours", "Days"}."Minutes") -> ("Triggered?"=w243:bool)  [unwired: 1 in]
                n139 = local read "FP Data"() -> (w233:sgl[])
                n140 = Or(x=w241, y=w244) -> (x .or. y?=w231:bool)
                n141 = Or(x=w241, y=w243) -> (x .or. y?=w242:bool)
                n142 = And(x=w242, y=w250) -> (x .and. y?=w261:bool)
                n143 = And(x=w231, y=w249) -> (x .and. y?=w232:bool)
                n144 = case shown="True" w232 {
                  tunnel: w233 -> [_ w288]
                  tunnel: w234 -> [_ w301]
                  tunnel: w236 -> [_ w300]
                  tunnel: w235 -> [_ w302]
                  tunnel: "Log Options" -> [_ w295]
                  tunnel: w241 -> [_ _]
                  tunnel: w239 -> [_ w282]
                  frame False {
                  }
                  frame True {
                    n145 = Unbundle By Name(w295) -> ("Filename suffix"=w292:string, "AVS_Path 2"=w294:path, "AVS_FName"=w293:string, "NewFevery"=w286:u32, "Time Units"=w285:enum16{"Minutes", "Hours", "Days"}, "Date Format"=w284:string)
                    n146 = call "Combine Data 4 logging.vi"("FP Status Bits"=w300, "Time Format String"=w284, "PT2 Data"=w282, "PT1 Data"=w302, "MG Data"=w301, "FP Data"=w288) -> ("Array"=w291:string[])  [unwired: 1 in]
                    n147 = local read "Cur Path"() -> (w289:path)
                    n148 = call "Format header.vi"("FP Data"=w288) -> ("Header string"=w287:string)  [unwired: 4 in]
                    n149 = call "File Date.vi"("Cur Path"=w289) -> ("Time Stamp"=w299:timestamp)  [unwired: 4 in]
                    n150 = call "Time Elapsed time.vi"("Time Units"=w285, "Delay Time"=w286, "Time Old In"=w299) -> ("T>dT?"=w290:bool)  [unwired: 2 out]
                    n151 = case shown="True" w290 {
                      tunnel: [w304 w306] -> w297
                      tunnel: [_ w310] -> w296
                      tunnel: w294 -> [_ w309]
                      tunnel: w293 -> [_ w308]
                      tunnel: w292 -> [_ w307]
                      tunnel: w289 -> [w304 _]
                      tunnel: w287 -> [_ w305]
                      frame False {
                      }
                      frame True {
                        n152 = call "GeneratePaths.vi"("Filename Suffix"=w307, "AVS_Path"=w309, "AVS_FName"=w308) -> ("Generated Log path"=w306:path)  [unwired: 11 in, 1 out]
                        n153 = Write to Text File(file (use dialog)=w306, text=w305) -> (error out=w310:errorcluster)  [unwired: 2 in, 2 out]
                      }
                    }
                    n154 = call "Write To Spreadsheet File (string) w Error.vi"("append to file? (new file:F)"=TRUE, "error in"=w296, "1D data"=w291, "file path (dialog if empty)"=w297) -> ("new file path (Not A Path if cancelled)"=→"Cur Path":path)  [unwired: 6 in, 1 out]
                    n155 = local write "ForceSave"(FALSE ("ForceSave")) -> ()
                  }
                }
                n156 = case shown="True" w261 {
                  tunnel: w234 -> [_ w271]
                  tunnel: w233 -> [_ w281]
                  tunnel: w235 -> [_ w272]
                  tunnel: w239 -> [_ w265]
                  frame False {
                  }
                  frame True {
                    w264 = 1 ("Smoothing window")
                    n157 = Get Date/Time In Seconds() -> (seconds since 1Jan1904=w280:timestamp)
                    n158 = To Double Precision Float(number=w280) -> (double precision float=w279:dbl)
                    n159 = call "AppendData1.vi"("Smoothing window"=w264, "Current Measurement"=w279) -> ("Data Out"=w262:dbl[])  [unwired: 4 in]
                    n160 = call "AppendData.vi"("Smoothing window"=w264, "Current Measurement"=w265) -> ("Data Out"=w263:sgl[][])  [unwired: 4 in]
                    n161 = call "AppendData.vi"("Smoothing window"=w264, "Current Measurement"=w281) -> ("Data Out"=w267:sgl[][])  [unwired: 4 in]
                    n162 = call "AppendData.vi"("Smoothing window"=w264, "Current Measurement"=w271) -> ("Data Out"=w268:sgl[][])  [unwired: 4 in]
                    n163 = call "AppendData.vi"("Smoothing window"=w264, "Current Measurement"=w272) -> ("Data Out"=w269:sgl[][])  [unwired: 4 in]
                    n164 = call "MultiRPlot_Select1.vi"("Time"=w262, "FP Plots Select"="FP Plots Select", "Data In"=w267) -> ("Out Array"=→"Front Panel":cluster{"Time":dbl[], "Value":dbl[]}[])  [unwired: 1 in]
                    n165 = call "MultiRPlot_Select1.vi"("Time"=w262, "FP Plots Select"="MG Plots Select", "Data In"=w268) -> ("Out Array"=→"MaxiGauge":cluster{"Time":dbl[], "Value":dbl[]}[])  [unwired: 1 in]
                    n166 = call "MultiRPlot_Select1.vi"("Time"=w262, "FP Plots Select"="PT1 Plots Select", "Data In"=w269) -> ("Out Array"=→"PT1 Status 2":cluster{"Time":dbl[], "Value":dbl[]}[])  [unwired: 1 in]
                    n167 = call "MultiRPlot_Select1.vi"("Time"=w262, "FP Plots Select"="PT2 Plots Select", "Data In"=w263) -> ("Out Array"=→"PT2 Status":cluster{"Time":dbl[], "Value":dbl[]}[])  [unwired: 1 in]
                  }
                }
                n168 = Array To Cluster(array=w233) -> (cluster=w260:T27)
                n169 = property on="P8" class="Ring (strict)"() -> ("Value"=w258:u16)  [unwired: 2 in, 2 out]
                n170 = Unbundle(w260) -> ("FP Data[0]"=→"P1" →"P1":sgl, "FP Data[1]"=→"P2" →"P2":sgl, "FP Data[2]"=→"P3" →"P3":sgl, "FP Data[3]"=→"P4" →"P4":sgl, "FP Data[4]"=→"P5" →"P5":sgl, "FP Data[5]"=→"P6" →"4He":sgl, "FP Data[6]"=→"P7" →"3He":sgl, "FP Data[7]"=→"Flow" →"FLOW":sgl, "FP Data[8]"=→"PC" →"PC":sgl)
                n171 = Index Array(array=w234, index=w258) -> (element=→"Pstill (P8)":dbl)
              }
              frame #1 {
                # "Flag from previous case: only log if true"
                n172 = case shown="True" w311 {
                  frame False {
                  }
                  frame True {
                    n173 = local read "FP Status bits"() -> (w314:u32[])
                    n174 = local read "MG Data"() -> (w317:dbl[])
                    n175 = local read "PT1 Data"() -> (w318:dbl[])
                    n176 = local read "FP Data"() -> (w316:sgl[])
                    n177 = local read "Mode"() -> (w313:u16)
                    n178 = Bundle By Name(cluster=T26 {"FP Data"=[], "MG Data"=[], "PT Data"=[], "FP Status Bits"=[], "Mode"=0} ("FP cluster"), "FP Data"=w316, "MG Data"=w317, "PT Data"=w318, "FP Status Bits"=w314, "Mode"=w313) -> (w315:T26)
                    n179 = call "FP to PGSQL.vi"("FP cluster"=w315) -> ()  [unwired: 10 in, 1 out]
                  }
                }
              }
              frame #2 {
                # "Check if the structure is \nnot empty and only one\nof Scalar or Array controls \nis set"
                # "Set FP control value from external script/program"
                n180 = local read "SetControl"() -> (w330:T7)
                n181 = Unbundle By Name(w330) -> ("Name"=w328:string, "Scalar"=w329:string, "Array"=w320:string[][])
                n182 = call "Empty 2D Array (String)__ogtk.vi"("Array"=w320) -> ("Empty Array?"=w323:bool)  [unwired: 8 in]
                n183 = Empty String/Path?(string/path=w328) -> (empty?=w324:bool)
                n184 = Empty String/Path?(string/path=w329) -> (empty?=w325:bool)
                n185 = Not(x=w324) -> (.not. x?=w326:bool)
                n186 = Not(x=w325) -> (.not. x?=w322:bool)
                n187 = Not(x=w323) -> (.not. x?=w319:bool)
                n188 = Exclusive Or(1:w319, 2:w322) -> (0:w321:bool)
                n189 = And(x=w326, y=w321) -> (x .and. y?=w327:bool)
                n190 = case shown="True" w327 {
                  tunnel: w328 -> [_ w334]
                  tunnel: w329 -> [_ w333]
                  tunnel: w320 -> [_ w332]
                  tunnel: w319 -> [_ w331]
                  frame False {
                  }
                  frame True {
                    n191 = flat-sequence {
                      tunnel: w334 -> [w338]
                      tunnel: w333 -> [w337]
                      tunnel: w332 -> [w335]
                      tunnel: w331 -> [w336]
                      frame #0 {
                        n192 = local read "VIRef"() -> (w339:T1)
                        n193 = case shown="True" w336 {
                          tunnel: w339 -> [w342 w345]
                          tunnel: w338 -> [w341 w344]
                          tunnel: w337 -> [w340 _]
                          tunnel: w335 -> [_ w343]
                          frame False {
                            n194 = call "Push2VI.vi"("New Value"=w340, "element"=w341, "VIRef"=w342) -> ()  [unwired: 8 in, 1 out]
                          }
                          frame True {
                            n195 = call "PushArray2VI.vi"("Str"=w343, "element"=w344, "VIRef"=w345) -> ()  [unwired: 8 in, 1 out]
                          }
                        }
                      }
                      frame #1 {
                        w347 = ""
                        # "Empty the cluster to flag that\nthe command is processed"
                        n196 = Bundle(w347, w347, "Array"=string[][] []) -> (→"SetControl":cluster{string, string, "Array":string[][]})  [unwired: 1 in]
                      }
                    }
                  }
                }
              }
              frame #3 {
                n197 = local read "MG error"() -> (w353:errorcluster)
                n198 = local read "FP error"() -> (w354:errorcluster)
                n199 = Not(x=w354) -> (.not. x?=w352:bool)
                n200 = Not(x=w353) -> (.not. x?=w351:bool)
                n201 = Compound Arithmetic op=AND(w352, w351, "EnableAutoCond") -> (w349:bool)
                n202 = case shown="True" w349 {
                  tunnel: w356 -> [w357 w373]
                  tunnel: [w357 w372] -> w355
                  frame False {
                    n203 = call "MGI Milliseconds Since Last Reset.vi"("Reset (F)"=TRUE) -> ()  [unwired: 5 in, 2 out]
                  }
                  frame True {
                    n204 = local read "MG Data"() -> (w380:dbl[])
                    n205 = Index Array(array=w380, index="MG  channel") -> (element=w378:dbl)
                    n206 = Not(x="Cond2") -> (.not. x?=w374:bool)
                    n207 = Less?(x=w378, y="P threshold") -> (x < y?=w376:bool)
                    n208 = Or(x=w376, y=w374) -> (x .or. y?=w360:bool)
                    "SP reached? 3" <- w360
                    n209 = Not(x=w360) -> (.not. x?=w362:bool)
                    n210 = call "MGI Milliseconds Since Last Reset.vi"("Reset (F)"=w362) -> ("ms"=w371:u32)  [unwired: 5 in, 1 out]
                    n211 = Divide(x=w371, y=u32 1000) -> (x/y=w368:dbl)
                    "Delay Timer" <- w368
                    n212 = Multiply(x="Delay Time", y=u32 60) -> (x*y=w364:u32)
                    n213 = Not(x="Cond1") -> (.not. x?=w365:bool)
                    n214 = Greater Or Equal?(x=w368, y=w364) -> (x >= y?=w367:bool)
                    n215 = Or(x=w367, y=w365) -> (x .or. y?=w361:bool)
                    "SP reached? 2" <- w361
                    n216 = And(x=w360, y=w361) -> (x .and. y?=w359:bool)
                    "SP reached?" <- w359
                    n217 = case shown="True" w359 {
                      tunnel: w373 -> [w381 w383]
                      tunnel: [w381 w382] -> w372
                      frame False {
                      }
                      frame True {
                        # "Auto"
                        # "Start"
                        # "Reset"
                        n218 = call "BP togglekey.vi"("keynumber"=u16 10, "FrontPanel port"=w383) -> ("error out"=w395:T18, "FrontPanel port"=w390:refnum<visa-resource-name>)  [unwired: 2 in]
                        n219 = local write "EnableAutoCond"(FALSE ("EnableAutoCond")) -> ()
                        n220 = call "MGI Wait (U32).vi"("ms"=u32 2000, "Error In"=w395) -> ("Error Out"=w394:errorcluster)  [unwired: 5 in]
                        n221 = call "BP togglekey.vi"("error in"=w394, "keynumber"=u16 48, "FrontPanel port"=w390) -> ("error out"=w393:T18, "FrontPanel port"=w392:refnum<visa-resource-name>)  [unwired: 1 in]
                        n222 = call "MGI Wait (U32).vi"("ms"=u32 500, "Error In"=w393) -> ("Error Out"=w391:errorcluster)  [unwired: 5 in]
                        n223 = call "BP togglekey.vi"("error in"=w391, "keynumber"=u16 54, "FrontPanel port"=w392) -> ("FrontPanel port"=w382:refnum<visa-resource-name>)  [unwired: 1 in, 1 out]
                      }
                    }
                  }
                }
              }
            }
          }
          frame True {
            n224 = stacked-sequence {
              frame #0 {
                w404 = T28."Page Disabled & Grayed" ("Page Enabled State")
                w405 = u8 2 ("Disabled")
                w417 = u8 1 ("Disabled")
                w421 = u32 16777062
                w426 = u32 65382
                w425 = u32 0
                w424 = 0.1
                w423 = 2000
                w422 = 0
                n225 = property class="App"() -> ("App.Kind"=w427:T29)  [unwired: 2 in, 2 out]
                n226 = property on="Hide side panel" class="Bool (strict)"("Val(Sgnl)"=FALSE ("Value (Signaling)")) -> ()  [unwired: 2 in, 2 out]
                n227 = property on="S1" class="TabCtl (strict)"("Disabled"=w405) -> ()  [unwired: 2 in, 2 out]
                n228 = property on="S2" class="TabCtl (strict)"("Disabled"=w405) -> ()  [unwired: 2 in, 2 out]
                n229 = property on="Stop" class="Bool (strict)"("Disabled"=w405) -> ()  [unwired: 2 in, 2 out]
                n230 = property on="Error panel" class="TabCtl (strict)"("Disabled"=w405) -> ()  [unwired: 2 in, 2 out]
                n231 = property on="Main Panel" class="TabCtl (strict)"("Disabled"=w405) -> ()  [unwired: 2 in, 2 out]
                n232 = property on="Main Panel" class="TabCtl (strict)"("Disabled"=w405) -> ()  [unwired: 2 in, 2 out]
                n233 = call "Current VIs Reference__ogtk.vi"() -> ("Current VI's reference"=w411:refnum<vi>)  [unwired: 5 in]
                n234 = case shown="\"Run Time System\"" w427 {
                  tunnel: [w429 w438] -> w428
                  frame "invalid app kind", Default {
                    n235 = control-ref of="This VI"() -> (w430:refnum<vi>)
                    n236 = property class="VI"(reference=w430) -> ("Hist.Revision"=w431:u32)  [unwired: 1 in, 2 out]
                    n237 = Divide(x=w431, y=1000.0 ("x")) -> (x/y=w435:dbl)
                    n238 = Number To Fractional String(use system decimal point (T)=FALSE, number=w435, precision (6)=i16 2) -> (F-format string=w436:string)  [unwired: 1 in]
                    n239 = Concatenate Strings("" ("string"), w436) -> (w429:string)
                  }
                  frame "Run Time System" {
                    n240 = call <userlib>:"MGI Get Executable Version.vi"() -> ("Version"=w438:string)  [unwired: 7 in]
                  }
                }
                "V" <- w428
                n241 = local write "Cur Path"(path "") -> ()
                n242 = call "GetFrontPanelControls.vi"("Ref to VI"=w411) -> ("VIRef"=w412:T1)  [unwired: 9 in, 1 out]
                "VIRef" <- w412
                n243 = Unbundle By Name(w412) -> ("Full Name"=→"ControlNames":string[])
                n244 = call "Current VI's Path__ogtk.vi"() -> ("Current VI's Path (+ Relative)"=w398:path)  [unwired: 1 in]
                n245 = property on="Side Panel" class="TabCtl (strict)"("Value"=enum32{"Main", "Settings", "Advanced"}."Settings" ("Side Panel")) -> ("Pages"=w401:refnum<vi>[])  [unwired: 2 in, 2 out]
                n246 = Path To String(path=w398) -> (string=→"VI path":string)
                n247 = Index Array(array=w401) -> (element #1=w402:refnum<vi>, element #3=w403:refnum<vi>)  [unwired: 3 in, 1 out]
                n248 = property class="Page"(reference=w402, "PageEnb"=w404) -> ()  [unwired: 1 in, 2 out]
                n249 = property class="Page"(reference=w403, "PageEnb"=w404) -> ()  [unwired: 1 in, 2 out]
                n250 = property on="3He" class="Slide (strict)"("Scale.Range:Minimum"=w422, "Scale.Range:Maximum"=w423, "Scale.Range:Increment"=w424) -> ()  [unwired: 2 in, 2 out]
                n251 = property on="P1" class="DigNum (strict)"("Numeric Text.Text Colors:Text Color"=w425, "Numeric Text.Text Colors:BG Color"=w421) -> ()  [unwired: 2 in, 2 out]
                n252 = property on="P4" class="DigNum (strict)"("Numeric Text.Text Colors:Text Color"=w425, "Numeric Text.Text Colors:BG Color"=w426) -> ()  [unwired: 2 in, 2 out]
                n253 = Initialize Array(FALSE, 64 ("dimension size")) -> (w397:bool[])
                n254 = property on="Start" class="Bool (strict)"("Visible"=TRUE, "Disabled"=u8 0) -> ()  [unwired: 2 in, 2 out]
                n255 = control-ref of="LEDs"() -> (w408:refnum<vi>)
                n256 = call "FP Set Binking Controls.vi"("Cluster in"=w408, "Array of blinking states"=w397, "Array of relais states"=w397) -> ()  [unwired: 13 in]
                n257 = property on="P2" class="DigNum (strict)"("Numeric Text.Text Colors:Text Color"=w425, "Numeric Text.Text Colors:BG Color"=w421) -> ()  [unwired: 2 in, 2 out]
                n258 = property on="P5" class="DigNum (strict)"("Numeric Text.Text Colors:Text Color"=w425, "Numeric Text.Text Colors:BG Color"=w426) -> ()  [unwired: 2 in, 2 out]
                n259 = property on="4He" class="Slide (strict)"("Scale.Range:Minimum"=w422, "Scale.Range:Maximum"=w423, "Scale.Range:Increment"=w424) -> ()  [unwired: 2 in, 2 out]
                n260 = control-ref of="LEDs 2"() -> (w409:refnum<vi>)
                n261 = property on="Configuration" class="Clust (strict)"("Disabled"=u8 0) -> ()  [unwired: 2 in, 2 out]
                n262 = call "FP Set Binking Controls.vi"("Cluster in"=w409, "Array of blinking states"=w397, "Array of relais states"=w397) -> ()  [unwired: 13 in]
                n263 = local write "EnableAutoCond"(FALSE ("EnableAutoCond")) -> ()
                n264 = property on="P3" class="DigNum (strict)"("Numeric Text.Text Colors:Text Color"=w425, "Numeric Text.Text Colors:BG Color"=w421) -> ()  [unwired: 2 in, 2 out]
                n265 = property on="FLOW" class="DigNum (strict)"("Numeric Text.Text Colors:Text Color"=w425, "Numeric Text.Text Colors:BG Color"=w426) -> ()  [unwired: 2 in, 2 out]
                n266 = property on="Panel ID" class="Str"("Text.Text Colors:Text Color"=u32 13311) -> ()  [unwired: 2 in, 2 out]
                n267 = property on="Buttons" class="Clust"("Disabled"=w417) -> ()  [unwired: 2 in, 2 out]
                n268 = property on="Buttons 2" class="Clust"("Disabled"=w417) -> ()  [unwired: 2 in, 2 out]
              }
              frame #1 {
                # "First load the settings from the old location then \nfrom the new one. This way the program will \"transfer\" \nthe settings to the new config file after the upgrade"
                n269 = call "Create Dir if Non-Existant__ogtk.vi"("Directory Path"=path "C:/LC Data/Configuration/FP" ("Relative path (.)")) -> ("dup Directory Path"=w441:path)  [unwired: 8 in, 2 out]
                n270 = call "Build Path - Traditional__ogtk.vi"("name or relative path"="FP config.ini", "base path"=w441) -> ("appended path"=w439:path)
                n271 = control-ref of="Configuration"() -> (w451:refnum<vi>)
                n272 = control-ref of="ADC scaling"() -> (w448:refnum<vi>)
                n273 = control-ref of="Log Options"() -> (w447:refnum<vi>)
                n274 = call "Current VIs Parent Directory__ogtk.vi"("Relative path (.)"=path "config.ini") -> ("Parent Directory (+ Relative)"=w449:path)  [unwired: 4 in]
                n275 = Build Array(w451, w448, w447) -> (w444:refnum<vi>[])
                n276 = call "Save Load Settings to File by Ref with path.vi"("Array of Cluster References"=w444, "Action"=enum8{"Load", "Save"}."Load", "Configuration file"=w449) -> ("error out"=w445:errorcluster)  [unwired: 6 in]
                n277 = call "MGI Clear Error.vi"("Error In"=w445) -> ("Error Out"=w446:errorcluster)  [unwired: 6 in]
                n278 = call "Save Load Settings to File by Ref with path.vi"("Array of Cluster References"=w444, "Action"=enum8{"Load", "Save"}."Load", "error in (no error)"=w446, "Configuration file"=w439) -> ()  [unwired: 5 in, 1 out]
              }
            }
          }
        }
      }
      event "Start": Value Change {
        n279 = event-data() -> ()  [unwired: 1 in, 6 out]
        n280 = stacked-sequence {
          tunnel: w465 -> [_ w515 _ _ _ _]
          tunnel: [_ w514 _ _ _ _] -> w464
          tunnel: w463 -> [w480 _ _ _ _ _]
          tunnel: [w467 _ _ _ _ _] -> w462
          tunnel: w461 -> [_ _ _ _ _ w613]
          tunnel: w460 -> [_ _ _ w586 _ _]
          tunnel: w459 -> [_ _ _ w585 _ _]
          tunnel: [_ _ _ w583 _ _] -> w458
          tunnel: [_ _ _ w584 _ _] -> w457
          tunnel: w453 -> [_ _ _ _ _ _]
          tunnel: w456 -> [_ _ _ _ _ _]
          tunnel: [_ _ w541 _ _ _] -> w455
          tunnel: [_ _ w545 _ _ _] -> w454
          frame #0 {
            n281 = call "Stop Display Busy AE.vi"("Action"=enum16{"Write", "Read"}."Write", "Error In"=T18 {"error"=FALSE, "code"=0, "source"=""} ("error in"), "Stop?"=FALSE) -> ("Error Out"=w468:errorcluster)  [unwired: 7 in, 1 out]
            n282 = property on="FP baud rate" class="DigNum (strict)"() -> ("Value"=w479:u32)  [unwired: 2 in, 2 out]
            n283 = call "FP-Scan ports.vi"("Error in"=w468, "baud rate"=w479, "RS232 port"=w480) -> ("Error out"=w471:errorcluster, "ID string"=w477:string, "VISA Refnum out"=w478:refnum<visa-resource-name>)  [unwired: 5 in, 1 out]
            "Panel ID" <- w477
            n284 = call "Stop Display Busy AE.vi"("Action"=enum16{"Write", "Read"}."Write", "Error In"=w471, "Stop?"=TRUE) -> ("Error Out"=w470:errorcluster)  [unwired: 7 in, 1 out]
            n285 = call "Get GHS version and type.vi"("ID string"=w477, "error in (no error)"=w470) -> ("Panel Version"=w485:bool, "System Type"=w484:bool, "error out"=w481:errorcluster)  [unwired: 4 in]
            n286 = call "Display Busy.vi"("error in (no error)"=w468, "Title"="Trying to connect to the Front Panel") -> ()  [unwired: 8 in, 2 out]
            n287 = Boolean To (0,1)(Boolean=w485) -> (0, 1=w466:i16)
            n288 = Boolean To (0,1)(Boolean=w484) -> (0, 1=w483:i16)
            n289 = property on="FP Layout" class="TabCtl (strict)"("Value"=w466) -> ()  [unwired: 2 in, 2 out]
            n290 = property on="Panel Layout" class="Enum (strict)"("Value"=w466) -> ()  [unwired: 2 in, 2 out]
            n291 = property on="Type" class="RadioBtnsControl (strict)"("Val(Sgnl)"=w483) -> ()  [unwired: 2 in, 2 out]
            n292 = call "BP query settings.vi"("error in"=w481, "FrontPanel port"=w478) -> ("error out"=w482:T18, "array of 4 x 16 bit unsigned"=w492:u16[], "FrontPanel port"=w493:refnum<visa-resource-name>)  [unwired: 2 in, 1 out]
            "FP error" <- w482
            n293 = call "BP query P5.vi"("error in"=w482, "FrontPanel port"=w493) -> ("error out"=w506:T18, "array of 2 x 16 bit unsigned"=w511:u16[], "FrontPanel port"=w512:refnum<visa-resource-name>)  [unwired: 2 in, 1 out]
            n294 = Array To Cluster(array=w492) -> (cluster=w491:T30)
            n295 = Array To Cluster(array=w511) -> (cluster=w504:T31)
            n296 = call "Disable on error.vi"("error out"=w506) -> ("Numeric"=w507:i16)
            n297 = property on="P6&7 limits" class="Clust (strict)"("Value"=w491) -> ()  [unwired: 2 in, 2 out]
            n298 = call "BP query NCP5.vi"("error in"=w482, "FrontPanel port"=w512) -> ("error out"=w509:T18, "array of 3 x 16 bit unsigned"=w510:u16[], "FrontPanel port"=w503:refnum<visa-resource-name>)  [unwired: 2 in, 1 out]
            n299 = property on="P5 Settings" class="Clust (strict)"("Value"=w504, "Disabled"=w507) -> ()  [unwired: 2 in, 2 out]
            n300 = Array To Cluster(array=w510) -> (cluster=w505:T32)
            n301 = call "Disable on error.vi"("error out"=w509) -> ("Numeric"=w508:i16)
            n302 = call "BP query NCP5B.vi"("error in"=w482, "FrontPanel port"=w503) -> ("error out"=w500:T18, "array of 3 x 16 bit unsigned"=w501:u16[], "FrontPanel port"=w502:refnum<visa-resource-name>)  [unwired: 2 in, 1 out]
            n303 = property on="NCP5 Settings" class="Clust (strict)"("Value"=w505, "Disabled"=w508) -> ()  [unwired: 2 in, 2 out]
            n304 = Array To Cluster(array=w501) -> (cluster=w498:cluster{"array of 3 x 16 bit unsigned[0]":u16})
            n305 = property on="P6&7 Settings" class="Clust (strict)"("Value"=w491) -> ()  [unwired: 2 in, 2 out]
            n306 = call "Disable on error.vi"("error out"=w500) -> ("Numeric"=w499:i16)
            n307 = call "BP Query REC.vi"("error in"=w482, "FrontPanel port"=w502) -> ("error out"=w496:T18, "array of 3 x 16 bit unsigned"=w497:u16[], "FrontPanel port"=w490:refnum<visa-resource-name>)  [unwired: 2 in, 1 out]
            n308 = property on="P5 limits" class="Clust (strict)"("Value"=w504) -> ()  [unwired: 2 in, 2 out]
            n309 = property on="NCP5B Settings" class="Clust (strict)"("Value"=w498, "Disabled"=w499) -> ()  [unwired: 2 in, 2 out]
            n310 = Array To Cluster(array=w497) -> (cluster=w494:T32)
            n311 = call "Disable on error.vi"("error out"=w496) -> ("Numeric"=w495:i16)
            n312 = call "BP Query Turbo.vi"("error in"=w482, "FrontPanel port"=w490) -> ("error out"=w488:T18, "array of 3 x 16 bit unsigned"=w487:u16[], "FrontPanel port"=w467:refnum<visa-resource-name>)  [unwired: 2 in, 1 out]
            "FP port" <- w467
            n313 = property on="REC Settings" class="Clust (strict)"("Value"=w494, "Disabled"=w495) -> ()  [unwired: 2 in, 2 out]
            n314 = property on="NCP5 limits" class="Clust (strict)"("Value"=w505) -> ()  [unwired: 2 in, 2 out]
            n315 = Array To Cluster(array=w487) -> (cluster=w486:cluster{"array of 3 x 16 bit unsigned[0]":u16})
            n316 = call "Disable on error.vi"("error out"=w488) -> ("Numeric"=w489:i16)
            n317 = property on="S1&2 Settings" class="Clust (strict)"("Value"=w486, "Disabled"=w489) -> ()  [unwired: 2 in, 2 out]
            n318 = property on="NCP5B limits" class="Clust (strict)"("Value"=w498) -> ()  [unwired: 2 in, 2 out]
            n319 = property on="REC limits" class="Clust (strict)"("Value"=w494) -> ()  [unwired: 2 in, 2 out]
            n320 = property on="FP port number" class="VISAName"("Value"=w467) -> ()  [unwired: 2 in, 2 out]
            n321 = property on="S1&2 limits" class="Clust (strict)"("Value"=w486) -> ()  [unwired: 2 in, 2 out]
          }
          frame #1 {
            w517 = T18 {"error"=FALSE, "code"=0, "source"=""}  # No error
            n322 = property on="MG Enabled?" class="Bool (strict)"() -> ("Value"=w516:bool)  [unwired: 2 in, 2 out]
            n323 = case shown="True" w516 {
              tunnel: [w520 w537] -> w513
              tunnel: [w518 w521] -> w514
              tunnel: w517 -> [w520 w527]
              tunnel: [FALSE TRUE] -> _
              tunnel: w515 -> [w518 w532]
              frame False {
                # "MaxiGauge not connected"
              }
              frame True {
                n324 = call "Stop Display Busy AE.vi"("Action"=enum16{"Write", "Read"}."Write", "Error In"=w527, "Stop?"=FALSE) -> ("Error Out"=w522:errorcluster)  [unwired: 7 in, 1 out]
                n325 = call "MG- Scan ports.vi"("Error in"=w522, "RS232 port"=w532) -> ("Error out"=w524:errorcluster, "ID string"=→"Maxigauge ID":string, "VISA Refnum out"=w531:refnum<visa-resource-name>)  [unwired: 6 in, 1 out]
                n326 = call "Stop Display Busy AE.vi"("Action"=enum16{"Write", "Read"}."Write", "Error In"=w524, "Stop?"=TRUE) -> ()  [unwired: 7 in, 2 out]
                n327 = call "Display Busy.vi"("error in (no error)"=w522, "Title"="Trying to connect to the MaxiGauge") -> ()  [unwired: 8 in, 2 out]
                n328 = call "MG Get Channels Labels.vi"("MaxiGauge port"=w531) -> ("Array"=w535:string[], "MaxiGauge port"=w521:refnum<visa-resource-name>, "error out"=w537:errorcluster)  [unwired: 1 in]
                "MG port" <- w521
                n329 = Array To Cluster(array=w535) -> (cluster=→"Cluster":T33)
                n330 = for {
                  tunnel: w535 -> [w539] mode=indexing
                  i -> [w540]
                  n331 = property on="MaxiGauge" class="XYGraph (strict)"("Active Plot"=w540, "Plot.Plot Name"=w539) -> ()  [unwired: 2 in, 2 out]
                }
                n332 = Search 1D Array(1D array=w535, element="STIL") -> (index of element=w533:i32)  [unwired: 1 in]
                n333 = property on="MG  channel P8" class="Ring (strict)"("Value"=w533) -> ()  [unwired: 2 in, 2 out]
                n334 = property on="MG port number" class="VISAName"("Value"=w521) -> ()  [unwired: 2 in, 2 out]
              }
            }
            "MG error" <- w513
          }
          frame #2 {
            n335 = property on="PT1 port \nnumber" class="VISAName"() -> ("Value"=w544:refnum<visa-resource-name>)  [unwired: 2 in, 2 out]
            n336 = property on="PT1 Enabled?" class="Bool (strict)"() -> ("Value"=w550:bool)  [unwired: 2 in, 2 out]
            n337 = case shown="True" w550 {
              tunnel: w544 -> [_ w582]
              tunnel: [u16 0 ("Port Number out") w581] -> w541
              tunnel: [errorcluster {"status"=FALSE, "code"=0, "source"=""} ("Error out") w573] -> w549
              tunnel: [refnum<visa-resource-name> refnum ("VISA Refnum out") w570] -> w542
              frame False {
              }
              frame True {
                n338 = call "Stop Display Busy AE.vi"("Action"=enum16{"Write", "Read"}."Write", "Stop?"=FALSE) -> ("Error Out"=w571:errorcluster)  [unwired: 8 in, 1 out]
                n339 = property on="PT1 Bauds" class="DigNum (strict)"() -> ("Value"=w580:u32)  [unwired: 2 in, 2 out]
                n340 = property on="PT1 Address" class="DigNum (strict)"() -> ("Value"=w579:u8)  [unwired: 2 in, 2 out]
                n341 = call "PT-Scan ports.vi"("Error in"=w571, "PT Address"=w579, "Baud rate"=w580, "RS232 port"=w582) -> ("Error out"=w574:errorcluster, "Port Number out"=w581:u16, "serial Port out"=w570:refnum<visa-resource-name>)  [unwired: 3 in, 2 out]
                n342 = call "Display Busy.vi"("error in (no error)"=w571, "Title"="Trying to connect to PulseTube1") -> ()  [unwired: 8 in, 2 out]
                n343 = property on="PT1 port \nnumber" class="VISAName"("Value"=w570) -> ()  [unwired: 2 in, 2 out]
                n344 = call "Stop Display Busy AE.vi"("Action"=enum16{"Write", "Read"}."Write", "Error In"=w574, "Stop?"=TRUE) -> ("Error Out"=w573:errorcluster)  [unwired: 7 in, 1 out]
              }
            }
            "PT1 error" <- w549
            "PT1 port" <- w541
            n345 = property on="PT2 port \nnumber" class="VISAName"() -> ("Value"=w543:refnum<visa-resource-name>)  [unwired: 2 in, 2 out]
            n346 = property on="PT2 Enabled?" class="Bool (strict)"() -> ("Value"=w547:bool)  [unwired: 2 in, 2 out]
            n347 = Build Array(w542) -> (w548:refnum<visa-resource-name>[])
            n348 = case shown="True" w547 {
              tunnel: w543 -> [_ w566]
              tunnel: [u16 0 ("Port Number out") w565] -> w545
              tunnel: [errorcluster {"status"=FALSE, "code"=0, "source"=""} ("Error out") w554] -> w546
              tunnel: w548 -> [_ w562]
              frame False {
              }
              frame True {
                n349 = call "Stop Display Busy AE.vi"("Action"=enum16{"Write", "Read"}."Write", "Stop?"=FALSE) -> ("Error Out"=w558:errorcluster)  [unwired: 8 in, 1 out]
                n350 = property on="PT2 Bauds" class="DigNum (strict)"() -> ("Value"=w564:u32)  [unwired: 2 in, 2 out]
                n351 = property on="PT2 Address" class="DigNum (strict)"() -> ("Value"=w563:u8)  [unwired: 2 in, 2 out]
                n352 = call "PT-Scan ports.vi"("RS232 ports to skip"=w562, "Error in"=w558, "PT Address"=w563, "Baud rate"=w564, "RS232 port"=w566) -> ("Error out"=w555:errorcluster, "Port Number out"=w565:u16, "serial Port out"=w553:refnum<visa-resource-name>)  [unwired: 2 in, 2 out]
                n353 = call "Display Busy.vi"("error in (no error)"=w558, "Title"="Trying to connect to PulseTube2") -> ()  [unwired: 8 in, 2 out]
                n354 = property on="PT2 port \nnumber" class="VISAName"("Value"=w553) -> ()  [unwired: 2 in, 2 out]
                n355 = call "Stop Display Busy AE.vi"("Action"=enum16{"Write", "Read"}."Write", "Error In"=w555, "Stop?"=TRUE) -> ("Error Out"=w554:errorcluster)  [unwired: 7 in, 1 out]
              }
            }
            "PT2 error" <- w546
            "PT2 port" <- w545
          }
          frame #3 {
            n356 = disable-structure shown="Disabled" {
              disable-tunnel: w586 -> [w592 w600]
              disable-tunnel: w585 -> [w591 w599]
              disable-tunnel: [w590 w599] -> w584
              disable-tunnel: [w587 w600] -> w583
              frame Disabled {
                n357 = property on="S2 Enabled?" class="Bool (strict)"() -> ("Value"=w588:bool)  [unwired: 2 in, 2 out]
                n358 = property on="S1 Enabled?" class="Bool (strict)"() -> ("Value"=w589:bool)  [unwired: 2 in, 2 out]
                n359 = case shown="False" w589 {
                  tunnel: w592 -> [w596 w598]
                  tunnel: [w596 w597] -> w587
                  frame False {
                  }
                  frame True {
                    n360 = call "PV Initialize.vi"("VISA session in"=w598) -> ("VISA session out"=w597:refnum<visa-resource-name>)  [unwired: 9 in, 1 out]
                  }
                }
                n361 = case shown="False" w588 {
                  tunnel: w591 -> [w593 w595]
                  tunnel: [w593 w594] -> w590
                  frame False {
                  }
                  frame True {
                    n362 = call "PV Initialize.vi"("VISA session in"=w595) -> ("VISA session out"=w594:refnum<visa-resource-name>)  [unwired: 9 in, 1 out]
                  }
                }
              }
              frame Enabled {
              }
            }
          }
          frame #4 {
            w602 = T28."Page Enabled" ("Page Enabled State")
            w607 = u8 0 ("Disabled")
            w610 = u8 0 ("Disabled")
            n363 = property on="Configuration" class="Clust (strict)"("Disabled"=u8 2) -> ()  [unwired: 2 in, 2 out]
            n364 = property on="Buttons" class="Clust"("Disabled"=w610) -> ()  [unwired: 2 in, 2 out]
            n365 = property on="Buttons 2" class="Clust"("Disabled"=w610) -> ()  [unwired: 2 in, 2 out]
            n366 = local write "Start"(FALSE ("Start")) -> ()
            n367 = property on="Main Panel" class="TabCtl (strict)"("Disabled"=w607) -> ()  [unwired: 2 in, 2 out]
            n368 = property on="Main Panel" class="TabCtl (strict)"("Disabled"=w607) -> ()  [unwired: 2 in, 2 out]
            n369 = property on="Stop" class="Bool (strict)"("Disabled"=w607) -> ()  [unwired: 2 in, 2 out]
            n370 = property on="Error panel" class="TabCtl (strict)"("Disabled"=w607) -> ()  [unwired: 2 in, 2 out]
            n371 = property on="Side Panel" class="TabCtl (strict)"("Value"=enum32{"Main", "Settings", "Advanced"}."Main" ("Side Panel")) -> ("Pages"=w604:refnum<vi>[])  [unwired: 2 in, 2 out]
            n372 = Index Array(array=w604) -> (element #1=w605:refnum<vi>, element #2=w601:refnum<vi>, element #3=w606:refnum<vi>)  [unwired: 3 in]
            n373 = property class="Page"(reference=w605, "PageEnb"=w602) -> ()  [unwired: 1 in, 2 out]
            n374 = property class="Page"(reference=w601, "PageEnb"=w602) -> ()  [unwired: 1 in, 2 out]
            n375 = property class="Page"(reference=w606, "PageEnb"=w602) -> ()  [unwired: 1 in, 2 out]
          }
          frame #5 {
            n376 = Set Occurrence(w613) -> ()
            n377 = property on="Start" class="Bool (strict)"("Visible"=TRUE, "Disabled"=u8 2) -> ()  [unwired: 2 in, 2 out]
          }
        }
      }
      event "Stop": Value Change {
        w614 = u16 0 ("Port Number out")
        w615 = refnum<visa-resource-name> refnum ("PT port")
        n378 = event-data() -> ()  [unwired: 1 in, 6 out]
        n379 = call "Stop Display Busy AE.vi"("Action"=enum16{"Write", "Read"}."Write", "Stop?"=FALSE) -> ("Error Out"=w618:errorcluster)  [unwired: 8 in, 1 out]
        n380 = call "Display Busy.vi"("error in (no error)"=w618, "Title"="Stopping...") -> ()  [unwired: 8 in, 2 out]
        n381 = flat-sequence {
          tunnel: w625 -> [w632]
          tunnel: [w631] -> w620
          tunnel: w618 -> [w631]
          tunnel: w629 -> [w636]
          tunnel: w628 -> [w634]
          tunnel: w627 -> [w635]
          tunnel: w626 -> [w637]
          tunnel: [w633] -> w621
          tunnel: w620 -> [w633]
          tunnel: [w640] -> w622
          tunnel: w621 -> [w640]
          tunnel: w622 -> [w647]
          tunnel: [w646] -> w617
          tunnel: w617 -> [w652]
          tunnel: [w652] -> w616
          tunnel: w616 -> [_]
          frame #0 {
            n382 = Wait on Occurrence(2:w632) -> ()  [unwired: 2 in, 1 out]
          }
          frame #1 {
            n383 = VISA Close(VISA resource name=w636) -> ()  [unwired: 1 in, 1 out]
            n384 = VISA Close(VISA resource name=w634) -> ()  [unwired: 1 in, 1 out]
            n385 = VISA Close(VISA resource name=w635) -> ()  [unwired: 1 in, 1 out]
            n386 = VISA Close(VISA resource name=w637) -> ()  [unwired: 1 in, 1 out]
          }
          frame #2 {
            n387 = control-ref of="Configuration"() -> (w643:refnum<vi>)
            n388 = control-ref of="ADC scaling"() -> (w641:refnum<vi>)
            n389 = control-ref of="Log Options"() -> (w639:refnum<vi>)
            n390 = property on="Start" class="Bool (strict)"("Visible"=TRUE) -> ()  [unwired: 2 in, 2 out]
            n391 = Build Array(w643, w641, w639) -> (w644:refnum<vi>[])
            n392 = call "Save Load Settings to File by Ref with path.vi"("Array of Cluster References"=w644, "Action"=enum8{"Load", "Save"}."Save", "Configuration file"=path "C:/LC Data/Configuration/FP/FP config.ini" ("Relative path (.)")) -> ()  [unwired: 6 in, 1 out]
          }
          frame #3 {
            n393 = call "Stop Display Busy AE.vi"("Action"=enum16{"Write", "Read"}."Write", "Error In"=w647, "Stop?"=TRUE) -> ("Error Out"=w646:errorcluster)  [unwired: 7 in, 1 out]
            n394 = property on="Stop" class="Bool (strict)"("Value"=FALSE ("stop")) -> ()  [unwired: 2 in, 2 out]
          }
          frame #4 {
            n395 = Wait (ms)(milliseconds to wait=u32 500) -> ()  [unwired: 1 out]
          }
          frame #5 {
            n396 = Stop(stop? (T)=TRUE) -> ()
          }
        }
      }
      event "PT Start": Value Change {
        w662 = u16 54529 items=["Compressor START"=54529, "Compressor STOP"=50584, "Error Code"=26020, "Reset Max/Min"=54235] ("Command")
        n397 = event-data() -> ()  [unwired: 1 in, 6 out]
        n398 = property on="PT1 Address" class="DigNum (strict)"() -> ("Value"=w655:u8)  [unwired: 2 in, 2 out]
        n399 = property on="PT1 Bauds" class="DigNum (strict)"() -> ("Value"=w654:u32)  [unwired: 2 in, 2 out]
        n400 = call "PT Send Command.vi"("PT1 port"=w659, "PT Address"=w655, "PT Bauds"=w654, "Command"=w662) -> ()  [unwired: 1 in, 2 out]
      }
      event "PT Start 2": Value Change {
        w671 = u16 54529 items=["Compressor START"=54529, "Compressor STOP"=50584, "Error Code"=26020, "Reset Max/Min"=54235] ("Command")
        n401 = event-data() -> ()  [unwired: 1 in, 6 out]
        n402 = property on="PT2 Address" class="DigNum (strict)"() -> ("Value"=w664:u8)  [unwired: 2 in, 2 out]
        n403 = property on="PT2 Bauds" class="DigNum (strict)"() -> ("Value"=w663:u32)  [unwired: 2 in, 2 out]
        n404 = call "PT Send Command.vi"("PT1 port"=w665, "PT Address"=w664, "PT Bauds"=w663, "Command"=w671) -> ()  [unwired: 1 in, 2 out]
      }
      event "PT_stop": Value Change {
        w680 = u16 50584 items=["Compressor START"=54529, "Compressor STOP"=50584, "Error Code"=26020, "Reset Max/Min"=54235] ("Command")
        n405 = event-data() -> ()  [unwired: 1 in, 1 out]
        n406 = property on="PT1 Address" class="DigNum (strict)"() -> ("Value"=w673:u8)  [unwired: 2 in, 2 out]
        n407 = property on="PT1 Bauds" class="DigNum (strict)"() -> ("Value"=w672:u32)  [unwired: 2 in, 2 out]
        n408 = call "PT Send Command.vi"("PT1 port"=w677, "PT Address"=w673, "PT Bauds"=w672, "Command"=w680) -> ()  [unwired: 1 in, 2 out]
      }
      event "PT_stop 2": Value Change {
        w689 = u16 50584 items=["Compressor START"=54529, "Compressor STOP"=50584, "Error Code"=26020, "Reset Max/Min"=54235] ("Command")
        n409 = event-data() -> ()  [unwired: 1 in, 1 out]
        n410 = property on="PT2 Address" class="DigNum (strict)"() -> ("Value"=w682:u8)  [unwired: 2 in, 2 out]
        n411 = property on="PT2 Bauds" class="DigNum (strict)"() -> ("Value"=w681:u32)  [unwired: 2 in, 2 out]
        n412 = call "PT Send Command.vi"("PT1 port"=w683, "PT Address"=w682, "PT Bauds"=w681, "Command"=w689) -> ()  [unwired: 1 in, 2 out]
      }
      event "PT Error Code": Value Change {
        n413 = event-data() -> ("OldVal"=w698:i32, "NewVal"=w694:i32)  [unwired: 1 in]
        n414 = Not Equal?(x=w698, y=w694) -> (x != y?=w697:bool)
        n415 = global read "ErrCodeStatusLkup.vi" "Error code/name/description Firmware V1.5"() -> (w695:string)
        n416 = case shown="Default" w694 {
          tunnel: w696 -> [_ w709]
          frame 0, 14..23 {
            # "No Error or Warning"
            "Attempts Counter" <- u16 0 ("Attempts Counter")
          }
          frame Default {
            # "Error"
            n417 = local read "Attempts Counter"() -> (w715:u16)
            n418 = Less?(x=w715, y="Attempts") -> (x < y?=w712:bool)
            n419 = And(x=w712, y="Restart PT on Error?") -> (x .and. y?=w711:bool)
            n420 = case shown="True" w711 {
              tunnel: "Time delay" -> [_ w717]
              tunnel: w709 -> [_ w716]
              frame False {
              }
              frame True {
                n421 = flat-sequence {
                  tunnel: w716 -> [w718]
                  tunnel: w717 -> [w722]
                  frame #0 {
                    n422 = call "PT start.vi"("PT1 port"=w718) -> ()  [unwired: 1 in, 2 out]
                  }
                  frame #1 {
                    n423 = local read "Attempts Counter"() -> (w720:u16)
                    n424 = Increment(x=w720) -> (x+1=w719:u16)
                    n425 = local write "Attempts Counter"(w719) -> ()
                  }
                  frame #2 {
                    n426 = Multiply(x=w722, y=u16 1000) -> (x*y=w723:u16)
                    n427 = Wait (ms)(milliseconds to wait=w723) -> ()  [unwired: 1 out]
                  }
                }
              }
            }
          }
        }
        n428 = Pick Line(multi-line string=w695, line index=w694) -> (output string=w693:string)  [unwired: 1 in]
        "PT Error" <- w693
        n429 = case shown="True" w697 {
          tunnel: w694 -> [_ w704]
          tunnel: w693 -> [_ w701]
          frame False {
          }
          frame True {
            n430 = Format Date/Time String() -> (date/time string=w702:string)  [unwired: 3 in]
            n431 = Number To Decimal String(number=w704) -> (decimal integer string=w703:string)  [unwired: 1 in]
            n432 = Build Array(w702, w703, w701) -> (w705:string[])
            n433 = feedback #1() -> (w706:string[][])  [unwired: 1 in]
            "Error Log" <- w706
            n434 = Build Array (concatenate)(w706, w705) -> (w707:string[][])
            n435 = feedback-in #1(w707) -> ()
          }
        }
      }
      event "PT_ResetValues": Value Change {
        w732 = u16 54235 items=["Compressor START"=54529, "Compressor STOP"=50584, "Error Code"=26020, "Reset Max/Min"=54235] ("Command")
        n436 = event-data() -> ()  [unwired: 1 in, 1 out]
        n437 = property on="PT1 Address" class="DigNum (strict)"() -> ("Value"=w725:u8)  [unwired: 2 in, 2 out]
        n438 = property on="PT1 Bauds" class="DigNum (strict)"() -> ("Value"=w724:u32)  [unwired: 2 in, 2 out]
        n439 = call "PT Send Command.vi"("PT1 port"=w729, "PT Address"=w725, "PT Bauds"=w724, "Command"=w732) -> ()  [unwired: 1 in, 2 out]
      }
      event "PT_ResetValues 2": Value Change {
        w741 = u16 54235 items=["Compressor START"=54529, "Compressor STOP"=50584, "Error Code"=26020, "Reset Max/Min"=54235] ("Command")
        n440 = event-data() -> ()  [unwired: 1 in, 1 out]
        n441 = property on="PT2 Address" class="DigNum (strict)"() -> ("Value"=w734:u8)  [unwired: 2 in, 2 out]
        n442 = property on="PT2 Bauds" class="DigNum (strict)"() -> ("Value"=w733:u32)  [unwired: 2 in, 2 out]
        n443 = call "PT Send Command.vi"("PT1 port"=w735, "PT Address"=w734, "PT Bauds"=w733, "Command"=w741) -> ()  [unwired: 1 in, 2 out]
      }
      event "Buttons": Value Change {
        n444 = event-data() -> ("NewVal"=w750:T3)  [unwired: 1 in, 5 out]
        n445 = Cluster To Array(cluster=w750) -> (array=w749:bool[])
        n446 = while {
          tunnel: w749 -> [w754] mode=indexing
          tunnel: [w753] -> w748
          i -> [w753]
          stop <- w754 stop-if-true
        }
        n447 = Increment(x=w748) -> (x+1=w747:i32)
        n448 = call "BP togglekey.vi"("keynumber"=w747, "FrontPanel port"=w746) -> ("FrontPanel port"=w745:refnum<visa-resource-name>)  [unwired: 2 in, 1 out]
      }
      event "Buttons 2": Value Change {
        n449 = event-data() -> ("NewVal"=w763:T3)  [unwired: 1 in, 5 out]
        n450 = Cluster To Array(cluster=w763) -> (array=w762:bool[])
        n451 = while {
          tunnel: w762 -> [w767] mode=indexing
          tunnel: [w766] -> w761
          i -> [w766]
          stop <- w767 stop-if-true
        }
        n452 = Increment(x=w761) -> (x+1=w760:i32)
        n453 = call "BP togglekey.vi"("keynumber"=w760, "FrontPanel port"=w759) -> ("FrontPanel port"=w758:refnum<visa-resource-name>)  [unwired: 2 in, 1 out]
      }
      event "Button": Value Change {
        n454 = event-data() -> ()  [unwired: 1 in, 6 out]
        n455 = call "BP togglekey.vi"("keynumber"="Button", "FrontPanel port"=w773) -> ("FrontPanel port"=w772:refnum<visa-resource-name>)  [unwired: 2 in, 1 out]
      }
      event "SET VALUES": Value Change {
        n456 = event-data() -> ("OldVal"=w782:bool)  [unwired: 1 in, 5 out]
        n457 = property on="SET VALUES" class="Bool (strict)"("Value"=w782) -> ()  [unwired: 2 in, 2 out]
        n458 = stacked-sequence {
          tunnel: w777 -> [w788 w802 w817 w835 w850 w865]
          tunnel: [w784 _ _ _ _ _] -> w776
          frame #0 {
            n459 = local read "P6&7 Settings"() -> (w787:T13)
            n460 = local read "P6&7 limits"() -> (w786:T13)
            n461 = Not Equal?(x=w787, y=w786) -> (x != y?=w785:bool)
            n462 = case shown="True" w785 {
              tunnel: w788 -> [w790 w797]
              tunnel: [w790 w796] -> w784
              frame False {
                n463 = control-ref of="P6&7 Settings"() -> (w789:refnum<vi>)
                n464 = call "FP check parameters error.vi"("Clust Refnum"=w789) -> ()  [unwired: 6 in, 1 out]
              }
              frame True {
                n465 = control-ref of="P6&7 Settings"() -> (w793:refnum<vi>)
                n466 = call "BP Set Config.vi"("GHS Settings"="P6&7 Settings", "FrontPanel port"=w797) -> ("error out"=w795:T18, "FrontPanel port"=w801:refnum<visa-resource-name>)  [unwired: 2 in]
                n467 = call "FP check parameters error.vi"("error in"=w795, "Clust Refnum"=w793) -> ("error out"=w794:errorcluster)  [unwired: 5 in]
                n468 = call "BP query settings.vi"("error in"=w794, "FrontPanel port"=w801) -> ("error out"=w792:T18, "array of 4 x 16 bit unsigned"=w799:u16[], "BP response"=→"Panel response":string, "FrontPanel port"=w796:refnum<visa-resource-name>)  [unwired: 2 in]
                n469 = Array To Cluster(array=w799) -> (cluster=→"P6&7 limits":T30)
                n470 = local write "FP error"(w792) -> ()
              }
            }
          }
          frame #1 {
            n471 = local read "P5 Settings"() -> (w804:cluster{"P6 low":u16, "P6 high":u16})
            n472 = local read "P5 limits"() -> (w805:cluster{"P5 C1":u16, "P5 C2":u16})
            n473 = Not Equal?(x=w804, y=w805) -> (x != y?=w803:bool)
            n474 = case shown="True" w803 {
              tunnel: w802 -> [_ w812]
              frame False {
                n475 = control-ref of="P5 Settings"() -> (w806:refnum<vi>)
                n476 = call "FP check parameters error.vi"("Clust Refnum"=w806) -> ()  [unwired: 6 in, 1 out]
              }
              frame True {
                n477 = control-ref of="P5 Settings"() -> (w809:refnum<vi>)
                n478 = call "BP Set P5.vi"("P5 Settings"="P5 Settings", "FrontPanel port in"=w812) -> ("error out"=w816:errorcluster, "FrontPanel port out"=w815:refnum<visa-resource-name>)  [unwired: 2 in]
                n479 = call "FP check parameters error.vi"("error in"=w816, "Clust Refnum"=w809) -> ("error out"=w810:errorcluster)  [unwired: 5 in]
                n480 = call "BP query P5.vi"("error in"=w810, "FrontPanel port"=w815) -> ("error out"=w808:T18, "array of 2 x 16 bit unsigned"=w814:u16[], "BP response"=w807:string)  [unwired: 2 in, 1 out]
                n481 = Array To Cluster(array=w814) -> (cluster=→"P5 limits":T31)
                n482 = local write "Panel response"(w807) -> ()
                n483 = local write "FP error"(w808) -> ()
              }
            }
          }
          frame #2 {
            n484 = local read "NCP5 Settings"() -> (w819:T10)
            n485 = local read "NCP5 limits"() -> (w820:T12)
            n486 = Not Equal?(x=w819, y=w820) -> (x != y?=w818:bool)
            n487 = case shown="True" w818 {
              tunnel: w817 -> [_ w827]
              frame False {
                n488 = control-ref of="NCP5 Settings"() -> (w821:refnum<vi>)
                n489 = call "FP check parameters error.vi"("Clust Refnum"=w821) -> ()  [unwired: 6 in, 1 out]
              }
              frame True {
                n490 = control-ref of="NCP5 Settings"() -> (w824:refnum<vi>)
                n491 = call "BP Set NCP5.vi"("NCP5 Settings"="NCP5 Settings", "FrontPanel port in"=w827) -> ("error out"=w826:errorcluster, "FrontPanel port out"=w831:refnum<visa-resource-name>)  [unwired: 2 in]
                n492 = call "FP check parameters error.vi"("error in"=w826, "Clust Refnum"=w824) -> ("error out"=w825:errorcluster)  [unwired: 5 in]
                n493 = call "BP query NCP5.vi"("error in"=w825, "FrontPanel port"=w831) -> ("error out"=w823:T18, "array of 3 x 16 bit unsigned"=w829:u16[], "BP response"=w822:string)  [unwired: 2 in, 1 out]
                n494 = local write "Panel response"(w822) -> ()
                n495 = Array To Cluster(array=w829) -> (cluster=→"NCP5 limits":T32)
                n496 = local write "FP error"(w823) -> ()
              }
            }
          }
          frame #3 {
            n497 = local read "NCP5B Settings"() -> (w832:cluster{"P6 low":u16})
            n498 = local read "NCP5B limits"() -> (w833:cluster{"P5 NC4":u16})
            n499 = Not Equal?(x=w832, y=w833) -> (x != y?=w834:bool)
            n500 = case shown="True" w834 {
              tunnel: w835 -> [_ w842]
              frame False {
                n501 = control-ref of="NCP5B Settings"() -> (w836:refnum<vi>)
                n502 = call "FP check parameters error.vi"("Clust Refnum"=w836) -> ()  [unwired: 6 in, 1 out]
              }
              frame True {
                n503 = control-ref of="NCP5B Settings"() -> (w839:refnum<vi>)
                n504 = call "BP Set NCP5B.vi"("NCP5B"="NCP5B Settings", "FrontPanel port in"=w842) -> ("error out"=w841:errorcluster, "FrontPanel port out"=w843:refnum<visa-resource-name>)  [unwired: 2 in]
                n505 = call "FP check parameters error.vi"("error in"=w841, "Clust Refnum"=w839) -> ("error out"=w840:errorcluster)  [unwired: 5 in]
                n506 = call "BP query NCP5B.vi"("error in"=w840, "FrontPanel port"=w843) -> ("error out"=w838:T18, "array of 3 x 16 bit unsigned"=w844:u16[], "BP response"=w837:string)  [unwired: 2 in, 1 out]
                n507 = local write "Panel response"(w837) -> ()
                n508 = Array To Cluster(array=w844) -> (cluster=→"NCP5B limits":cluster{"array of 3 x 16 bit unsigned[0]":u16})
                n509 = local write "FP error"(w838) -> ()
              }
            }
          }
          frame #4 {
            n510 = local read "REC Settings"() -> (w848:T10)
            n511 = local read "REC limits"() -> (w849:T11)
            n512 = Not Equal?(x=w848, y=w849) -> (x != y?=w847:bool)
            n513 = case shown="True" w847 {
              tunnel: w850 -> [_ w857]
              frame False {
                n514 = control-ref of="REC Settings"() -> (w851:refnum<vi>)
                n515 = call "FP check parameters error.vi"("Clust Refnum"=w851) -> ()  [unwired: 6 in, 1 out]
              }
              frame True {
                n516 = control-ref of="REC Settings"() -> (w854:refnum<vi>)
                n517 = call "BP Set REC.vi"("NCP5 Settings"="REC Settings", "FrontPanel port in"=w857) -> ("error out"=w856:errorcluster, "FrontPanel port out"=w858:refnum<visa-resource-name>)  [unwired: 2 in]
                n518 = call "FP check parameters error.vi"("error in"=w856, "Clust Refnum"=w854) -> ("error out"=w855:errorcluster)  [unwired: 5 in]
                n519 = call "BP Query REC.vi"("error in"=w855, "FrontPanel port"=w858) -> ("error out"=w853:T18, "array of 3 x 16 bit unsigned"=w860:u16[], "BP response"=w852:string)  [unwired: 2 in, 1 out]
                n520 = local write "Panel response"(w852) -> ()
                n521 = Array To Cluster(array=w860) -> (cluster=→"REC limits":T32)
                n522 = local write "FP error"(w853) -> ()
              }
            }
          }
          frame #5 {
            n523 = local read "S1&2 Settings"() -> (w862:cluster{"Enum":enum16{"OFF", "ON"}})
            n524 = local read "S1&2 limits"() -> (w863:cluster{"S1&S2":enum16{"OFF", "ON"}})
            n525 = Not Equal?(x=w862, y=w863) -> (x != y?=w864:bool)
            n526 = case shown="True" w864 {
              tunnel: w865 -> [_ w874]
              frame False {
                n527 = control-ref of="S1&2 Settings"() -> (w866:refnum<vi>)
                n528 = call "FP check parameters error.vi"("Clust Refnum"=w866) -> ()  [unwired: 6 in, 1 out]
              }
              frame True {
                n529 = control-ref of="S1&2 Settings"() -> (w869:refnum<vi>)
                n530 = call "BP Set Turbo.vi"("S1&2 Settings"="S1&2 Settings", "FrontPanel port in"=w874) -> ("error out"=w871:errorcluster, "FrontPanel port out"=w875:refnum<visa-resource-name>)  [unwired: 2 in]
                n531 = call "FP check parameters error.vi"("error in"=w871, "Clust Refnum"=w869) -> ("error out"=w870:errorcluster)  [unwired: 5 in]
                n532 = call "BP Query Turbo.vi"("error in"=w870, "FrontPanel port"=w875) -> ("error out"=w868:T18, "array of 3 x 16 bit unsigned"=w876:u16[], "BP response"=w867:string)  [unwired: 2 in, 1 out]
                n533 = local write "Panel response"(w867) -> ()
                n534 = Array To Cluster(array=w876) -> (cluster=→"S1&2 limits":cluster{"array of 3 x 16 bit unsigned[0]":u16})
                n535 = local write "FP error"(w868) -> ()
              }
            }
          }
        }
      }
      event "Log Options.Plot data": Value Change {
        n536 = event-data() -> ("NewVal"=w883:bool)  [unwired: 1 in, 5 out]
        n537 = property on="Main Panel" class="TabCtl (strict)"() -> ("Pages"=w886:refnum<vi>[])  [unwired: 2 in, 2 out]
        n538 = Index Array(array=w886, index=2) -> (element=w884:refnum<vi>)
        n539 = property class="Page"(reference=w884, "PageVis"=w883) -> ()  [unwired: 1 in, 2 out]
      }
      event "Autoconf": Value Change {
        n540 = event-data() -> ()  [unwired: 1 in, 6 out]
      }
      event "Configuration": Value Change {
        n541 = event-data() -> ()  [unwired: 1 in, 6 out]
        n542 = VISA Close(VISA resource name=w904) -> ()  [unwired: 1 in, 1 out]
        n543 = VISA Close(VISA resource name=w905) -> ()  [unwired: 1 in, 1 out]
        n544 = VISA Close(VISA resource name=w902) -> ()  [unwired: 1 in, 1 out]
        n545 = VISA Close(VISA resource name=w900) -> ()  [unwired: 1 in, 1 out]
        n546 = Unbundle By Name("Configuration") -> ("PT1 port number"=w894:refnum<visa-resource-name>, "PT2 port number"=w896:refnum<visa-resource-name>, "FP port number"=w906:refnum<visa-resource-name>, "MG port number"=w903:refnum<visa-resource-name>, "S1 port"=w901:refnum<visa-resource-name>, "S2 port"=w899:refnum<visa-resource-name>)
        n547 = call "VISA to RS232 Port Nr.vi"("VISA Resource Name"=w894) -> ("Port Number"=w898:u8)  [unwired: 1 in]
        n548 = call "VISA to RS232 Port Nr.vi"("VISA Resource Name"=w896) -> ("Port Number"=w897:u8)  [unwired: 1 in]
        n549 = Increment(x=w898) -> (x+1=w893:u8)
        n550 = Increment(x=w897) -> (x+1=w895:u8)
      }
      event "Type": Value Change {
        n551 = event-data() -> ("NewVal"=w911:enum32{"Wet", "CF"})  [unwired: 1 in, 5 out]
        n552 = case shown="\"CF\", Default" w911 {
          tunnel: ["COMPRESSOR" ("Label.Text") "AUX 2" ("Label.Text")] -> w916
          tunnel: [TRUE ("Visible") FALSE ("Visible")] -> w912
          tunnel: ["From\nProbe" ("Text.Text") "From\nDewar" ("Text.Text")] -> w910
          tunnel: ["From\nOVC" ("Text.Text") "From\n1K pot" ("Text.Text")] -> w909
          frame "CF", Default {
          }
          frame "Wet" {
          }
        }
        n553 = property on="Main Panel" class="TabCtl (strict)"() -> ("Pages"=w915:refnum<vi>[])  [unwired: 2 in, 2 out]
        n554 = Index Array(array=w915, index=1) -> (element=w913:refnum<vi>)
        n555 = property on="COMPR/AUX 2" class="Bool (strict)"("Caption.Text"=w916) -> ()  [unwired: 2 in, 2 out]
        n556 = property on="String 3" class="Str"("Text.Text"=w910) -> ()  [unwired: 2 in, 2 out]
        n557 = property on="String" class="Str"("Text.Text"=w909) -> ()  [unwired: 2 in, 2 out]
        n558 = property on="BYPASS" class="Bool (strict)"("Visible"=w912) -> ()  [unwired: 2 in, 2 out]
        n559 = property on="PT STATUS" class="Bool (strict)"("Visible"=w912) -> ()  [unwired: 2 in, 2 out]
        n560 = property class="Page"(reference=w913, "PageVis"=w912) -> ()  [unwired: 1 in, 2 out]
        n561 = property on="String 4" class="Str"("Text.Text"=w910) -> ()  [unwired: 2 in, 2 out]
        n562 = property on="String 2" class="Str"("Text.Text"=w909) -> ()  [unwired: 2 in, 2 out]
      }
      event "Panel Layout": Value Change {
        n563 = event-data() -> ("NewVal"=w936:enum32{"OLD", "NEW"})  [unwired: 1 in, 5 out]
        n564 = property on="FP type" class="TabCtl (strict)"("Value"=w936) -> ()  [unwired: 2 in, 2 out]
      }
      event "FP Status bits": Value Change {
        n565 = event-data() -> ("OldVal"=w945:u32[], "NewVal"=w944:u32[])  [unwired: 1 in, 4 out]
        n566 = Not Equal?(x=w945, y=w944) -> (x != y?=w943:bool)
        n567 = case shown="True" w943 {
          frame False {
          }
          frame True {
            "ForceSave" <- TRUE ("ForceSave")
          }
        }
      }
      event "Front Panel", "MaxiGauge": Shortcut Menu Activation? {
        w951 = string[] ["Log Y"] ("item names")
        w963 = string[] ["Autoscale XY"] ("item names")
        n568 = event-data() -> ("MenuRef"=w949:refnum<k9>, "CtlRef"=w948:refnum<vi>)  [unwired: 1 in]
        n569 = Insert Menu Items(4:10, 7:w963, 8:w963, 9:w949) -> (3:w950:refnum<k9>)  [unwired: 2 in, 2 out]
        n570 = property class="XYGraph (strict)"(reference=w948) -> ("YScale.Mapping Mode"=w954:u8)  [unwired: 1 in, 2 out]
        n571 = Insert Menu Items(4:13, 7:w951, 8:w951, 9:w950) -> (3:w953:refnum<k9>)  [unwired: 2 in, 2 out]
        n572 = Not Equal To 0?(x=w954) -> (x != 0?=w955:bool)
        n573 = Set Menu Item Info(6:w955, 7:"Log Y", 11:w953) -> ()  [unwired: 4 in, 2 out]
        n574 = event-data() -> ()  [unwired: 2 in, 1 out]
      }
      event "Front Panel", "MaxiGauge": Shortcut Menu Selection (User) {
        n575 = event-data() -> ("CtlRef"=w967:refnum<vi>, "ItemTag"=w973:string)  [unwired: 1 in]
        n576 = Type Cast(type=refnum<vi> refnum ("R-Plot 0"), x=w967) -> (*(type *) &x=w966:refnum<vi>)
        n577 = case shown="\"Log Y\"" w973 {
          tunnel: w966 -> [_ w974 w976]
          frame Default {
          }
          frame "Autoscale XY" {
            w975 = u8 2 ("X Scale.Scale Fit")
            n578 = property class="XYGraph (strict)"(reference=w974, "XScale.ScaleFit"=w975, "YScale.ScaleFit"=w975) -> ()  [unwired: 1 in, 2 out]
          }
          frame "Log Y" {
            n579 = property class="XYGraph (strict)"(reference=w976) -> (reference out=w977:refnum<vi>, "YScale.Mapping Mode"=w978:u8)  [unwired: 1 in, 1 out]
            n580 = Equal To 0?(x=w978) -> (x = 0?=w979:bool)
            n581 = Boolean To (0,1)(Boolean=w979) -> (0, 1=w980:i16)
            n582 = property class="XYGraph (strict)"(reference=w977, "YScale.Mapping Mode"=w980) -> ()  [unwired: 1 in, 2 out]
          }
        }
      }
      event "Front Panel", "MaxiGauge": Scale Range Change {
        w988 = u8 0 ("X Scale.Scale Fit")
        n583 = event-data() -> ("CtlRef"=w987:refnum<vi>)  [unwired: 1 in, 7 out]
        n584 = property class="XYGraph (strict)"(reference=w987, "XScale.ScaleFit"=w988, "YScale.ScaleFit"=w988) -> ()  [unwired: 1 in, 2 out]
      }
      event "Reset Error": Value Change {
        n585 = event-data() -> ()  [unwired: 1 in, 6 out]
        n586 = property on="Device address S1" class="DigNum (strict)"() -> ("Value"=w991:u8)  [unwired: 2 in, 2 out]
        n587 = call "PV Error Reset.vi"("Adress of unit"=w991, "VISA session"=w996) -> ("VISA resource out"=w990:refnum<visa-resource-name>)  [unwired: 8 in, 1 out]
      }
      event "Reset Error 2": Value Change {
        n588 = event-data() -> ()  [unwired: 1 in, 6 out]
        n589 = property on="Device address S2" class="DigNum (strict)"() -> ("Value"=w999:u8)  [unwired: 2 in, 2 out]
        n590 = call "PV Error Reset.vi"("Adress of unit"=w999, "VISA session"=w1004) -> ("VISA resource out"=w998:refnum<visa-resource-name>)  [unwired: 8 in, 1 out]
      }
      event "Configuration.S1 Enabled?": Value Change {
        n591 = event-data() -> ("NewVal"=w1015:bool)  [unwired: 1 in, 5 out]
        n592 = Not(x=w1015) -> (.not. x?=w1014:bool)
        n593 = Boolean To (0,1)(Boolean=w1014) -> (0, 1=w1013:i16)
        n594 = Multiply(x=i16 2, y=w1013) -> (x*y=w1011:i16)
        n595 = property on="S1" class="TabCtl (strict)"("Disabled"=w1011) -> ()  [unwired: 2 in, 2 out]
      }
      event "Configuration.S2 Enabled?": Value Change {
        n596 = event-data() -> ("NewVal"=w1023:bool)  [unwired: 1 in, 5 out]
        n597 = Not(x=w1023) -> (.not. x?=w1026:bool)
        n598 = Boolean To (0,1)(Boolean=w1026) -> (0, 1=w1025:i16)
        n599 = Multiply(x=i16 2, y=w1025) -> (x*y=w1022:i16)
        n600 = property on="S2" class="TabCtl (strict)"("Disabled"=w1022) -> ()  [unwired: 2 in, 2 out]
      }
      event "Configuration.PT1 Enabled?", "Configuration.PT2 Enabled?": Value Change {
        n601 = event-data() -> ()  [unwired: 1 in, 6 out]
        n602 = property on="PT1 Enabled?" class="Bool (strict)"() -> ("Value"=w1028:bool)  [unwired: 2 in, 2 out]
        n603 = property on="PT2 Enabled?" class="Bool (strict)"() -> ("Value"=w1027:bool)  [unwired: 2 in, 2 out]
        n604 = property on="Main Panel" class="TabCtl (strict)"() -> ("Pages"=w1031:refnum<vi>[])  [unwired: 2 in, 2 out]
        n605 = Or(x=w1028, y=w1027) -> (x .or. y?=w1029:bool)
        n606 = Index Array(array=w1031) -> (element #2=w1030:refnum<vi>)  [unwired: 2 in, 1 out]
        n607 = property class="Page"(reference=w1030, "PageVis"=w1029) -> ()  [unwired: 1 in, 2 out]
      }
      event "Boolean 2": Value Change {
        n608 = event-data() -> ("NewVal"=w1044:bool)  [unwired: 1 in, 5 out]
        n609 = case shown="False" w1044 {
          frame True {
            n610 = property class="VI"() -> ("Front Panel.PanelBounds"=w1045:T34)  [unwired: 2 in, 2 out]
            n611 = Unbundle By Name(w1045) -> ("Left"=w1051:i16, "Top"=w1048:i16)
            n612 = Add(x=i16 955 ("right"), y=w1051) -> (x+y=w1050:i16)
            n613 = Add(x=w1048, y=i16 730) -> (x+y=w1046:i16)
            n614 = Bundle By Name(cluster=w1045, "Right"=w1050, "Bottom"=w1046) -> (w1052:T34)
            n615 = property class="VI"("Front Panel.PanelBounds"=w1052) -> ()  [unwired: 2 in, 2 out]
          }
          frame False {
            n616 = property class="VI"() -> ("Front Panel.PanelBounds"=w1053:T34)  [unwired: 2 in, 2 out]
            n617 = Unbundle By Name(w1053) -> ("Left"=w1059:i16, "Top"=w1056:i16)
            n618 = Add(x=i16 1259 ("right"), y=w1059) -> (x+y=w1058:i16)
            n619 = Add(x=w1056, y=i16 730) -> (x+y=w1054:i16)
            n620 = Bundle By Name(cluster=w1053, "Right"=w1058, "Bottom"=w1054) -> (w1060:T34)
            n621 = property class="VI"("Front Panel.PanelBounds"=w1060) -> ()  [unwired: 2 in, 2 out]
          }
        }
      }
      event "FP Plots Select", "MG Plots Select": Value Change {
        n622 = event-data() -> ()  [unwired: 1 in, 6 out]
        n623 = local write "ForceSave"(TRUE ("ForceSave")) -> ()
      }
      event "SendCMD": Value Change {
        n624 = event-data() -> ()  [unwired: 1 in, 6 out]
        n625 = call "BP Send Command.vi"("String"="Command", "FrontPanel port in"=w1071) -> ("string after ack"=→"Response":string, "FrontPanel port out"=w1070:refnum<visa-resource-name>)  [unwired: 1 in, 1 out]
      }
    }
  }
